vi "Scan.vi"() -> ()   [LabVIEW 2016]
doc: "Ce VI modèle est conçu pour le modèle de conception Gestionnaire de messages dans une file d'attente.\n\nLa boucle de gestion d'événements génère des messages en fonction des actions sur l'interface utilisateur.\n\nLa boucle de gestion de messages traite les messages générés par la boucle de gestion d'événements ou par d'autres messages. Les messages sont des valeurs chaîne ; il est donc facile d'ajouter de nouveaux messages à la structure condition Conditions de messages de la boucle de gestion de messages Chaque cluster Message peut en outre fournir une valeur optionnelle pour Données de message, un variant qui peut être converti aux données requises pour un message spécifique."
uses:
  controls/Enum.ctl
  controls/FPGAVIreferenceTypeDefScanEngine.ctl
  controls/ScanWaveform.ctl
  Course Project/support/Message Queue/Message Cluster.ctl
  <vilib>/Analysis/coordinate.llb/2D Cartesian Coordinate Rotation (Scalar).vi
  <vilib>/rvi/errors/niLvFpgaAdjustHostInterfaceError.vi
  <vilib>/rvi/interface/nirviReadWriteControl/nirviReadWriteControl.xnode
  FPGA Bitfiles/qnmController797_usbRIO_controllerFPGAmu.lvbitx
  <vilib>/regexp/Match Regular Expression.xnode
  Course Project/support/Message Queue/Message Queue.lvlib
  <vilib>/rvi/interface/nirviCloseFPGA/nirviCloseFPGA.xnode
  NiFpgaLv.dll
  <vilib>/Analysis/NI_AALPro.lvlib
  controls/FPGAVIreferenceTypeDef.ctl
  <vilib>/FPGAPlugInAG/USB-7856R OEM/niLvFpga_Close_USB-7856R OEM.vi
panel:
  out "String":string
  in  "Scan Parameters":enum32{"Scan Parameters"}(tab)
  in  "expno":u32
  in  "Exp Folder":string="<date>_exp<expno>"
  in  "Base Folder":path=path "C:/"
  in  "Slow scan axis":bool=TRUE
  out "Speed":dbl format="%#_3pm/s"
  in  "Speed":bool=TRUE
  in  "Lock Scan Lines":bool=TRUE
  in  "Lock Scan Height":bool=TRUE
  in  "Save now":bool
  in  "Auto Save":bool=TRUE
  in  "File name":string="test"
  in  "Scan Parameters":T1={"Width"=1e-09, "Height"=1e-09, "X Offset"=0.0, "Y Offset"=0.0, "Angle"=0.0, "Pixels"=256, "Lines"=256, "Time/Line"=1.0, "Scan Rate"=1.0} {"Scan Rate" format="%#_3pHz"; "Lines" min=2 max=8192 format="%#.0f"; "Pixels" min=2 max=8193 format="%#.0f"; "Height" format="%#.1pm"; "Width" format="%#.1pm"; "Angle" format="%.2f°"; "Y Offset" format="%#_4pm"; "X Offset" format="%#_4pm"; "Time/Line" format="%.2ps"}
  in  "Actions":T2
  # "Scan Parameters"
  # "Frame"
  # "Hz"
  # "s"
  # "Saving"
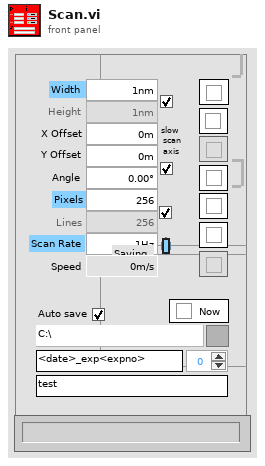
[diagram p1: front panel]
types:
  T1 = cluster{"Width":dbl, "Height":dbl, "X Offset":dbl, "Y Offset":dbl, "Angle":dbl, "Pixels":u16, "Lines":u16, "Time/Line":dbl, "Scan Rate":dbl}
  T2 = cluster{"Frame up":bool, "Frame down":bool, "Flip":bool, "Continuous":bool, "Pause":bool, "Stop":bool, "Move to center":bool}
  T3 = typedef "Message Queue.lvlib/All Message Queues.ctl" = cluster{"IU":refnum<queue>}
  T4 = typedef "Enum.ctl" = enum16{"Init", "Read", "Write"}
  T5 = cluster{"slowMoveWavePts":u16, "slowMoveAccelPts":u16, "moveSpeedSec":dbl}
  T6 = typedef "FPGAVIreferenceTypeDefScanEngine.ctl" = refnum<k20>
  T7 = enum32{"Bad", "Idle", "Run top level", "Running"}
  T8 = typedef "ScanWaveform.ctl" = enum16{"Sine", "Triangle", "Rounded"}
  T9 = cluster{"slowWavePts":u16, "fastWavePts":u16, "slowWaveType":T8, "fastWaveType":T8, "slowRoundPts":u16, "fastRoundPts":u16, "Update Parameters":bool, "Correct Hysteresis":bool, "UpdateFPGA":bool, "Update Graph":bool, "Hysteresis comp?":bool}
  T10 = enum8{"Enabled", "Disabled", "Disabled and Grayed Out"}
  T11 = cluster{"Sensitivity":cluster{"Sens X":dbl, "Sens Y":dbl, "Sens Z":dbl}, "Range":cluster{"Range X":dbl, "Range Y":dbl, "Range Z":dbl}, "HV gain":cluster{"HV gain X":dbl, "HV gain Y":dbl, "HV gain Z":dbl}}
  T12 = typedef "Message Queue.lvlib/Message Cluster.ctl" = cluster{"Message":string, "Données de message":variant}
  T13 = cluster{"slowWavePts":u16, "fastWavePts":u16, "slowWaveType":T8, "fastWaveType":T8, "slowRoundPts":u16, "fastRoundPts":u16, "singleDirectionScan":bool}
  T14 = cluster{"write":bool, "index":u16, "data":fxp<+/-,18,5>}
  T15 = cluster{"calibName":string[], "calibParameters":cluster{"Sensitivity":cluster{"Sens X":dbl, "Sens Y":dbl, "Sens Z":dbl}, "Range":cluster{"Range X":dbl, "Range Y":dbl, "Range Z":dbl}, "HV gain":cluster{"HV gain X":dbl, "HV gain Y":dbl, "HV gain Z":dbl}}[], "calibIndex":i32}
  T16 = cluster{"Sensitivity":cluster{"Sens X":dbl, "Sens Y":dbl, "Sens Z":dbl}, "Range":cluster{"Range X":dbl, "Range Y":dbl, "Range Z":dbl}, "HV gain":cluster{"HV gain X":dbl, "HV gain Y":dbl, "HV gain Z":dbl}}[]
  T17 = cluster{"scanEngineHz":u32, "feedbackHz":u32, "sicmHz":u32, "rampHz":u32}
  T18 = typedef "ScanParametersAllTypeDef.ctl" = cluster{"fastRoundPts":u16, "slowRoundPts":u16, "fastWaveType":T8, "slowWaveType":T8, "fastWavePts":u16, "slowWavePts":u16, "outputRateHz":u32, "yOffset":dbl, "xOffset":dbl, "scanSizeSlow":dbl, "scanSizeFast":dbl, "rotation":dbl, "timePerLine":dbl, "numLines":u16, "pointsPerLine":u32, "scanEnable":bool, "slowMoveWavePts":u16, "slowMoveAccelPts":u16, "moveSpeedSec":dbl, "singleDirectionScan":bool}
  T19 = cluster{"Width":dbl, "Height":dbl, "X Offset":dbl, "Y Offset":dbl, "Angle":dbl, "Pixels/Line":u16, "Lines":u16, "Time/Line":dbl, "Scan Rate":dbl}
  T20 = typedef "FPGAVIreferenceTypeDef.ctl" = refnum<k20>
  T21 = cluster{"fastScanSize":fxp<+,17,1>, "slowScanSize":fxp<+,17,1>, "invertSlowAxis":bool}
  T22 = cluster{"se.p.enable":bool, "se.p.singleDirection":bool, "se.p.haltScan":bool, "se.mot.p.start":bool}
  T23 = cluster{"startFwd":u16, "endFwd":u16, "startBwd":u16, "endBwd":u16, "disableBlanking":bool, "useFineCounter":bool}
  T24 = cluster{"Waveform Shape Fast In":dbl[], "Waveform Shape Slow In":dbl[]}
  T25 = cluster{"outputRate":u16, "fastDecFactor":u16, "outWaveSizeFast":u16, "pplUpsampling":u16, "numLines":u16, "se.p.fastInvDec":fxp<+,22,0>, "se.p.slowUpStep":fxp<+,28,0>, "se.p.outWaveSizeSlow":u16, "blankingMax":u32, "se.p.fastBlanking":cluster{"startFwd":u32, "endFwd":u32, "startBwd":u32, "endBwd":u32, "disableBlanking":bool, "useCoarseCounter":bool}}
  T26 = typedef "ScanWaveform.ctl" = enum16{"Sine Wave", "Triangle Wave", "Rounded Wave"}
  T27 = cluster{"slowWavePts":u16, "fastWavePts":u16, "slowWaveType":T26, "fastWaveType":T26, "slowRoundPts":u16, "fastRoundPts":u16, "Update Parameters":bool, "Correct Hysteresis":bool, "UpdateFPGA":bool, "Update Graph":bool, "Hysteresis comp?":bool}
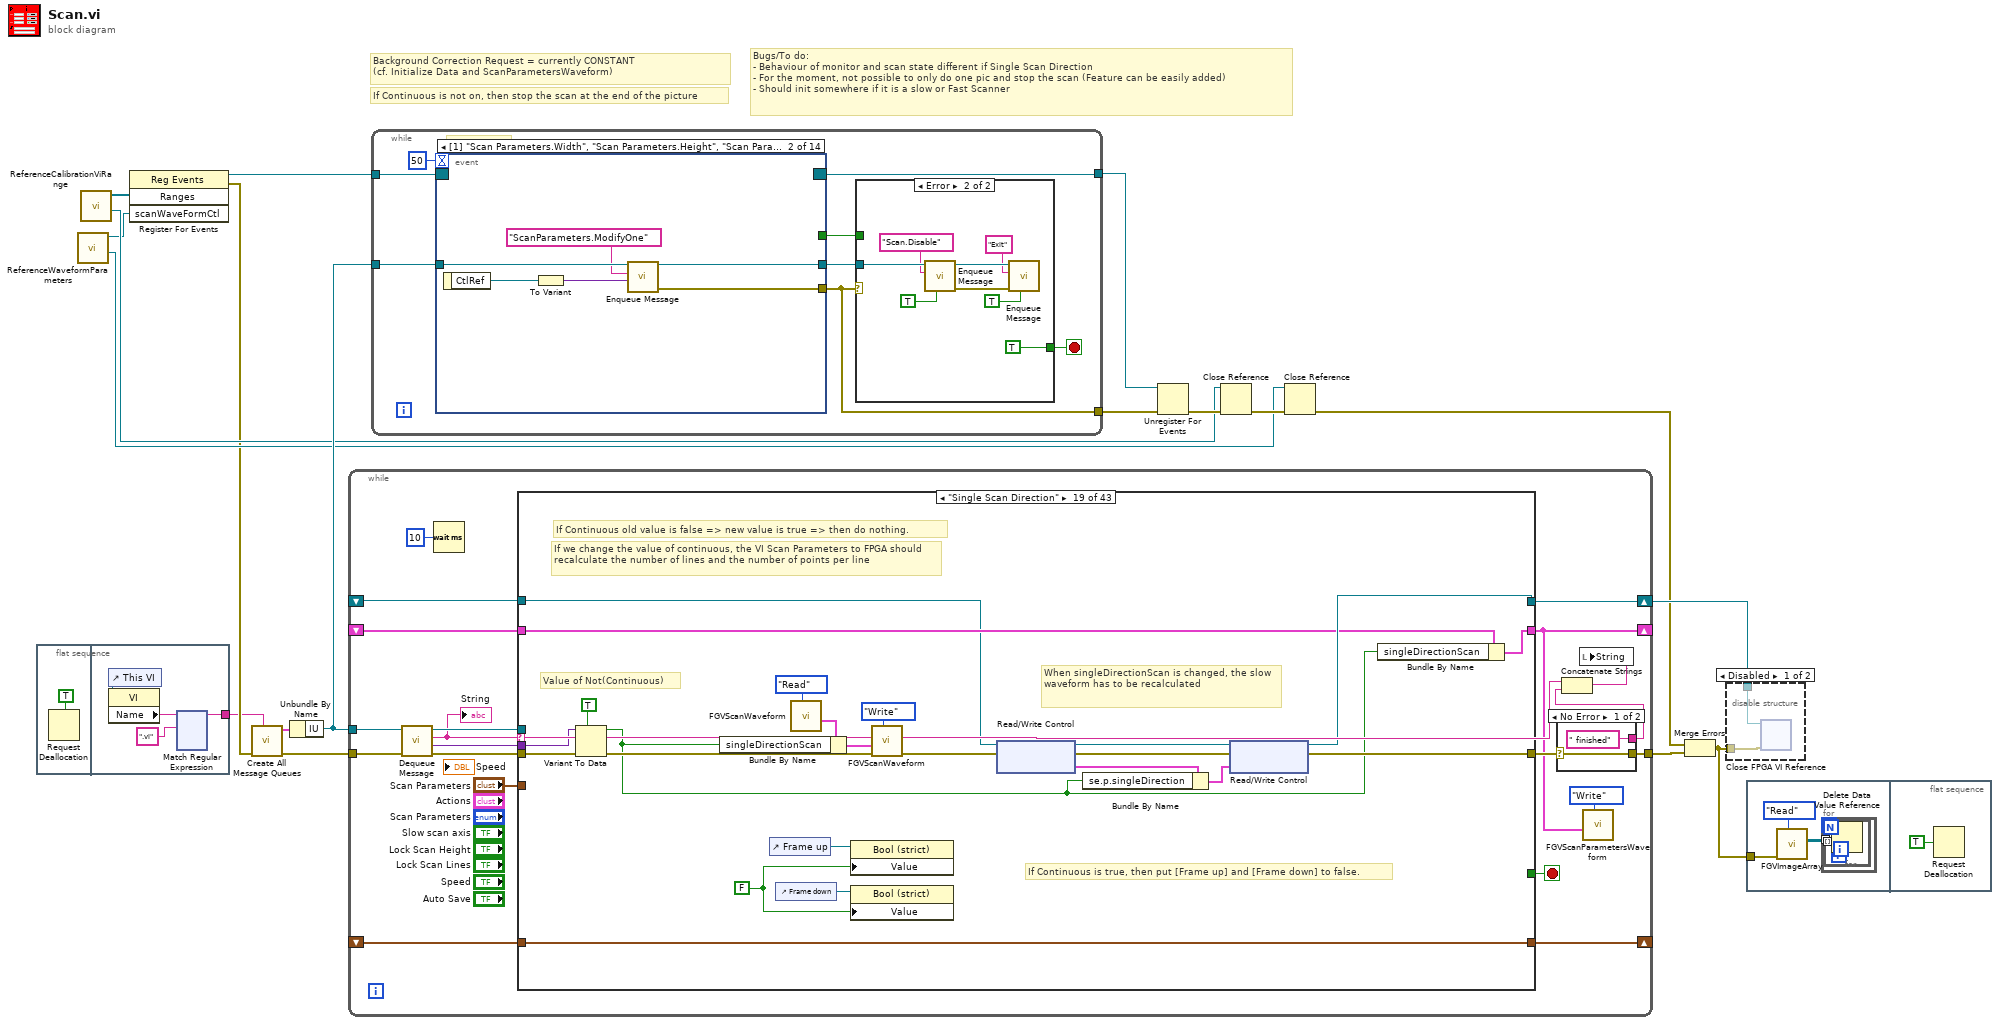
[diagram p0: block diagram]
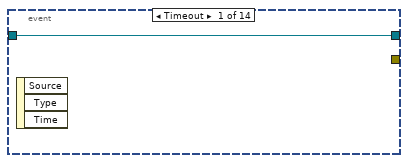
[diagram p4: hidden frame]
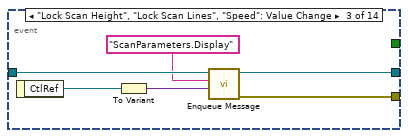
[diagram p5: hidden frame]
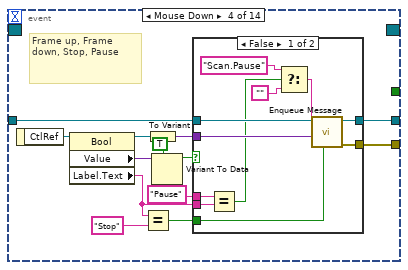
[diagram p6: hidden frame]
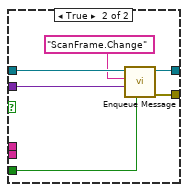
[diagram p7: hidden frame]
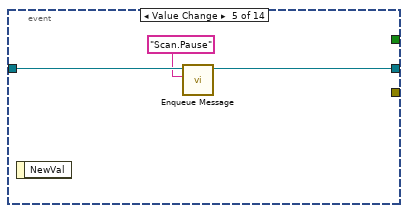
[diagram p8: hidden frame]
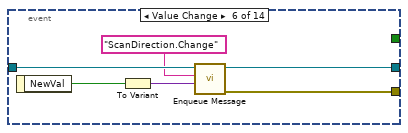
[diagram p9: hidden frame]
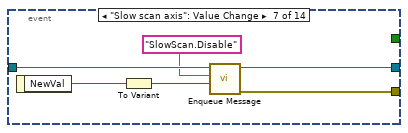
[diagram p10: hidden frame]
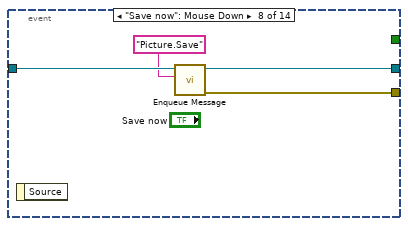
[diagram p11: hidden frame]
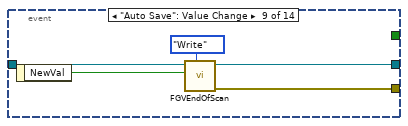
[diagram p12: hidden frame]
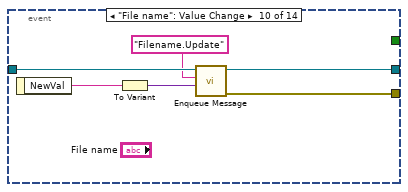
[diagram p13: hidden frame]
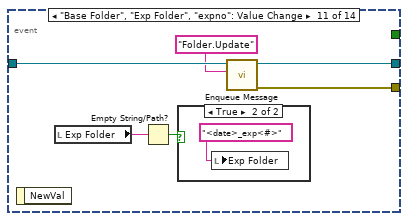
[diagram p14: hidden frame]
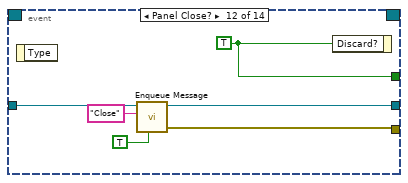
[diagram p16: hidden frame]
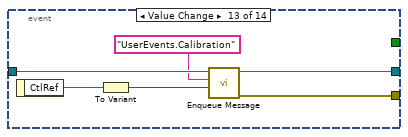
[diagram p17: hidden frame]
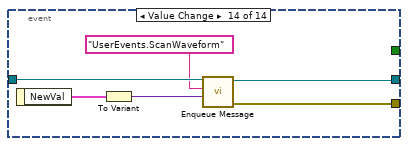
[diagram p18: hidden frame]
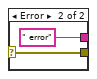
[diagram p19: hidden frame]
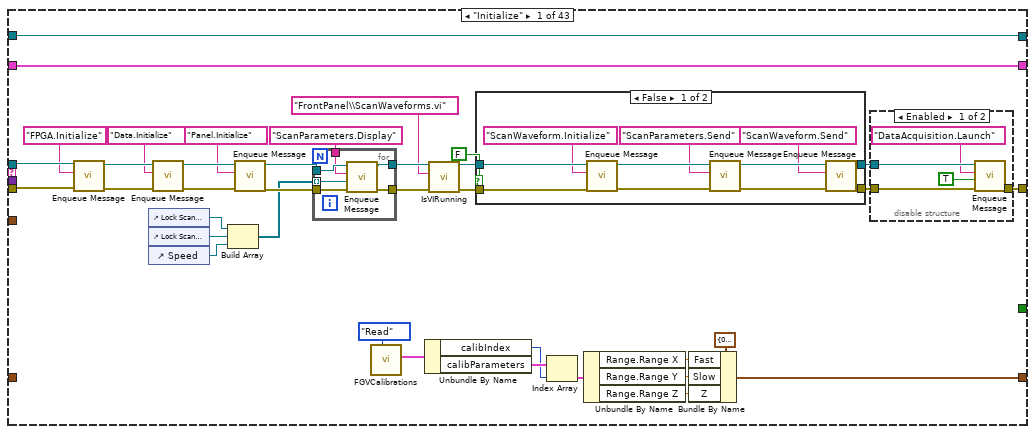
[diagram p20: hidden frame]
diagram:
  # "Bugs/To do:\n- Behaviour of monitor and scan state different if Single Scan Direction\n- For the moment, not possible to only do one pic and stop the scan (Feature can be easily added) \n- Should init somewhere if it is a slow or Fast Scanner"
  # "If Continuous is not on, then stop the scan at the end of the picture"
  # "Background Correction Request = currently CONSTANT\n(cf. Initialize Data and ScanParametersWaveform)"
  n1 = flat-sequence {
    tunnel: [w20] -> w2
    frame #0 {
      n2 = Request Deallocation(TRUE ("flag")) -> ()
    }
    frame #1 {
      n3 = control-ref of="This VI"() -> (w23:refnum<vi>)
      n4 = property class="VI"(reference=w23) -> ("Name"=w22:string)  [unwired: 1 in, 2 out]
      n5 = xnode "Match Regular Expression"("input string"=w22, "regular expression"=".vi") -> ("before match"=w20:string)  [unwired: 4 in, 4 out]
    }
  }
  n6 = call "ReferenceWaveformParameters.vi"() -> ("vi reference"=w5:refnum<vi>, "scanWaveFormCtl"=w7:refnum<vi>)  [unwired: 9 in, 1 out]
  n7 = call "ReferenceCalibrationViRange.vi"() -> ("vi reference"=w8:refnum<vi>, "Ranges"=w12:refnum<vi>[])  [unwired: 8 in, 2 out]
  n8 = register-events(w12, w7) -> (reference out=w11:refnum<event-registration>, error out=w3:errorcluster)  [unwired: 2 in]
  n9 = call "Create All Message Queues.vi"("QueueName"=w2, "ErrorIn"=w3) -> ("ErrorOut"=w18:errorcluster, "MessageQueueOut"=w17:T3)  [unwired: 8 in]
  n10 = Unbundle By Name(w17) -> ("IU"=w15:refnum<queue>)
  n11 = while {
    tunnel: w15 -> [w152]
    shift-right: [w142] -> _
    shift-left: _ -> [w138]
    shift-right: [w144] -> w13
    shift-left: _ -> [w151]
    tunnel: w18 -> [w156]
    tunnel: [w146] -> w16
    shift-right: [w140] -> _
    shift-left: _ -> [w139]
    stop <- w157 stop-if-true
    n12 = call "Dequeue Message.vi"("entrée d'erreur (pas d'erreur)"=w156, "File d'attente de messages"=w152) -> ("sortie d'erreur"=w155:errorcluster, "Données de message"=w154:variant, "Message"=w148:string, "File d'attente de message dup."=w153:refnum<queue>)  [unwired: 6 in]
    "String" <- w148
    n13 = Wait (ms)(milliseconds to wait=u32 10) -> ()  [unwired: 1 out]
    n14 = case "Conditions des messages" shown="\"Single Scan Direction\"" w148 {
      selector: w148 -> [_ _ _ _ _ _ _ _ _ _ _ _ _ _ _ _ _ _ _ _ _ _ _ _ _ _ _ _ _ _ _ _ _ _ _ _ _ _ _ _ _ _ w1429]
      tunnel: w153 -> [w193 _ _ _ _ w411 w430 w463 _ _ _ _ _ _ _ _ w598 w624 _ w739 _ _ w775 _ w880 _ w1114 _ _ _ _ _ _ _ w1312 _ w1342 _ _ _ _ _ _]
      tunnel: w155 -> [w185 w228 w265 w320 w338 w399 w429 w462 w490 w498 w511 w525 w536 w540 w555 w570 w585 w622 w719 w731 w748 w761 w774 w843 w878 w1078 w1108 w1148 w1157 w1162 w1192 w1238 w1272 w1292 w1323 w1330 w1338 w1360 w1373 w1393 w1397 w1405 _]
      tunnel: [w182 w237 w246 w302 w332 w400 w428 w453 w489 w495 w512 w525 w538 w554 w564 w570 w594 w619 w711 w729 w744 w761 w764 w856 w869 w1068 w1099 w1139 w1149 w1162 w1184 w1221 w1271 w1296 w1309 w1330 w1341 w1346 w1369 w1387 w1397 w1402 w1427] -> w147
      tunnel: [_ w239 _ _ _ _ TRUE _ _ _ _ _ _ _ _ _ _ _ _ _ _ _ _ _ _ _ _ _ _ _ _ _ _ _ _ _ _ _ _ _ _ _ _] -> w157
      tunnel: w154 -> [_ _ _ _ w335 _ _ w461 w488 _ _ _ w535 _ _ _ w582 w623 w721 w727 w747 _ w773 _ w879 w1077 w1110 _ _ _ _ _ _ _ _ _ w1336 _ _ _ _ w1404 _]
      tunnel: w138 -> [w190 w242 _ w321 w336 w397 w431 w456 w485 w497 w509 w523 w532 w551 w565 w568 w581 w613 w715 w725 w742 w759 w765 w852 w873 w1086 w1111 w1147 w1156 w1161 w1163 w1241 w1267 w1289 _ w1328 w1339 w1362 w1368 w1392 w1396 w1408 w1424]
      tunnel: [w190 w242 w253 w321 w336 w397 w431 w456 w474 w497 w509 w523 w532 w551 w565 w568 w581 w612 w710 w725 w742 w759 w763 w846 w866 w1070 w1111 w1147 w1156 w1161 w1163 w1241 w1267 w1289 w1313 w1328 w1339 w1343 w1368 w1380 w1396 w1408 w1424] -> w142
      tunnel: [w184 w225 w261 w322 w337 w403 w432 w457 w486 w496 w510 w524 w539 w552 w566 w569 w572 w615 w718 w726 w745 w760 w766 w850 w864 w1082 w1098 w1146 w1155 w1160 w1191 w1239 w1268 w1295 w1326 w1327 w1340 w1347 w1374 w1383 w1395 w1407 w1425] -> w144
      tunnel: w151 -> [w184 _ w261 w322 w337 w403 w432 w457 w486 w496 w510 w524 w539 w552 w566 w569 w573 w616 w705 w726 w746 w760 w766 w851 w865 w1087 w1098 w1146 w1155 w1160 w1170 w1240 w1269 w1294 w1326 w1327 w1340 w1361 w1375 w1388 w1395 w1407 w1425]
      tunnel: "Scan Parameters" -> [_ _ _ _ _ _ _ _ _ _ _ _ _ _ _ _ _ _ _ _ _ _ _ w848 _ w1080 _ _ _ _ _ _ _ _ _ _ _ _ _ _ _ _ _]
      tunnel: [w166 w241 w259 w324 w334 w396 w427 w439 w477 w491 w508 w522 w531 w550 w559 w567 w574 w626 w702 w723 w743 w758 w762 w844 w863 w1073 w1106 w1145 w1154 w1159 w1172 w1237 w1265 w1287 w1325 w1329 w1331 w1358 w1370 w1386 w1394 w1406 w1421] -> w140
      tunnel: w139 -> [_ w241 w259 w324 w334 w396 w427 _ w477 w491 w508 w522 w531 w550 w559 w567 w574 w626 w702 w723 w743 w758 w762 w844 w863 w1073 w1106 w1145 w1154 w1159 w1172 w1237 w1265 w1287 w1325 w1329 w1331 w1358 w1370 w1386 w1394 w1406 w1421]
      frame "Initialize" {
        n15 = call "Enqueue Message.vi"("error in"=w185, "Message"="FPGA.Initialize", "Queue"=w193) -> ("error out"=w189:errorcluster, "Queue dup."=w188:refnum<queue>)  [unwired: 7 in]
        n16 = control-ref of="Lock Scan Height"() -> (w179:refnum<vi>)
        n17 = control-ref of="Lock Scan Lines"() -> (w180:refnum<vi>)
        n18 = control-ref of="Speed"() -> (w181:refnum<vi>)
        n19 = call "Enqueue Message.vi"("error in"=w189, "Message"="Data.Initialize", "Queue"=w188) -> ("error out"=w186:errorcluster, "Queue dup."=w194:refnum<queue>)  [unwired: 7 in]
        n20 = Build Array(w179, w180, w181) -> (w178:refnum<vi>[])
        n21 = call "Enqueue Message.vi"("error in"=w186, "Message"="Panel.Initialize", "Queue"=w194) -> ("error out"=w197:errorcluster, "Queue dup."=w177:refnum<queue>)  [unwired: 7 in]
        n22 = for {
          tunnel: w177 -> [w222]
          tunnel: w178 -> [w221] mode=indexing
          tunnel: [w220] -> w164
          tunnel: w197 -> [w219]
          tunnel: [w218] -> w196
          tunnel: "ScanParameters.Display" ("Message") -> [w217]
          n23 = call "Enqueue Message.vi"("error in"=w219, "Data"=w221, "Message"=w217, "Queue"=w222) -> ("error out"=w220:errorcluster, "Queue dup."=w218:refnum<queue>)  [unwired: 6 in]
        }
        n24 = call "FGVCalibrations.vi"("Enum"=Enum."Read") -> ("calibOut"=w174:T15)  [unwired: 9 in, 1 out]
        n25 = Unbundle By Name(w174) -> ("calibIndex"=w169:i32, "calibParameters"=w173:T16)
        n26 = call "IsVIRunning.vi"("error in (no error)"=w164, "name or relative path"="FrontPanel\\ScanWaveforms.vi") -> ("error out"=w163:errorcluster)  [unwired: 8 in, 1 out]
        n27 = case shown="False" FALSE {
          tunnel: w196 -> [w208 w210]
          tunnel: [w207 w210] -> w195
          tunnel: [w199 w209] -> w183
          tunnel: w163 -> [w198 w209]
          frame False {
            n28 = call "Enqueue Message.vi"("error in"=w198, "Message"="ScanWaveform.Initialize", "Queue"=w208) -> ("error out"=w203:errorcluster, "Queue dup."=w204:refnum<queue>)  [unwired: 7 in]
            n29 = call "Enqueue Message.vi"("error in"=w203, "Message"="ScanParameters.Send", "Queue"=w204) -> ("error out"=w200:errorcluster, "Queue dup."=w206:refnum<queue>)  [unwired: 7 in]
            n30 = call "Enqueue Message.vi"("error in"=w200, "Message"="ScanWaveform.Send", "Queue"=w206) -> ("error out"=w199:errorcluster, "Queue dup."=w207:refnum<queue>)  [unwired: 7 in]
          }
          frame True {
          }
        }
        n31 = Index Array(array=w173, index=w169) -> (element=w170:T11)
        n32 = Unbundle By Name(w170) -> ("Range.Range X"=w172:dbl, "Range.Range Y"=w171:dbl, "Range.Range Z"=w168:dbl)
        n33 = Bundle By Name(cluster=cluster{"Slow":dbl, "Fast":dbl, "Z":dbl} {"Slow"=0.00015, "Fast"=0.00015, "Z"=0.00015} ("Calibration"), "Fast"=w172, "Slow"=w171, "Z"=w168) -> (w166:cluster{"Slow":dbl, "Fast":dbl, "Z":dbl})
        n34 = disable-structure shown="Enabled" {
          disable-tunnel: w195 -> [w215 _]
          disable-tunnel: w183 -> [w213 w216]
          disable-tunnel: [w212 w216] -> w182
          frame Enabled {
            n35 = call "Enqueue Message.vi"("error in"=w213, "Data"=TRUE, "Message"="DataAcquisition.Launch", "Queue"=w215) -> ("error out"=w212:errorcluster)  [unwired: 6 in, 1 out]
          }
          frame Disabled {
          }
        }
      }
      frame "FPGA.Initialize" {
        w224 = cluster{"outputRateHz":u32} {"outputRateHz"=800000}  # ioParams
        (unwired) T5 {"slowMoveWavePts"=1024, "slowMoveAccelPts"=128, "moveSpeedSec"=0.05}  # slowMoveParamsFast
        # "Scan engine output is clocked on base clock"
        # "1 : Scanner J slow\n0,2 : Scanner Fast"
        # "Initialize the Slow mouvment"
        # "ioParameters not Initialized"
        n36 = call "FGVfpgaAdressScanEngine.vi"("Enum"=Enum."Read", "error in"=w228) -> ("error out"=w236:errorcluster, "ioFreqHzOut"=w227:u32, "FPGA.SEout"=w226:T6)  [unwired: 5 in, 2 out]
        n37 = Equal?(x=w226, y=T6 refnum ("FPGAInterfaceOut")) -> (x = y?=w240:bool)
        n38 = Or(x=w236, y=w240) -> (x .or. y?=w239:bool)
        n39 = in-place {
          in-place-border: [w243] -> w230
          in-place-border: w227 -> [w245]
          n40 = in-place-cluster #1(w224) -> ("outputRateHz"=w244:u32)
          n41 = call "corerceFPGAClock.vi"("baseClock"=w245, "requestedFrequency"=w244) -> ("realFrequency"=w243:dbl)  [unwired: 7 in, 2 out]
          n42 = in-place-cluster #1("outputRateHz"=w243) -> (w223:cluster{"outputRateHz":u32})
        }
        n43 = call "FGVSamplingRates.vi"("Enum"=Enum."Read") -> ("samplingRatesOut"=w232:T17)  [unwired: 9 in, 1 out]
        n44 = Bundle By Name(cluster=w232, "scanEngineHz"=w230) -> (w231:T17)
        n45 = call "InitializeSmovement.vi"("error in"=w236, "slowMoveParams"=T5 {"slowMoveWavePts"=131, "slowMoveAccelPts"=30, "moveSpeedSec"=0.05}, "ioParams"=w223, "FPGAInterfaceIn"=w226) -> ("error out"=w237:errorcluster, "FPGAInterfaceOut"=w225:T6)  [unwired: 6 in]
        n46 = call "FGVSamplingRates.vi"("Enum"=Enum."Write", "samplingRatesIn"=w231) -> ()  [unwired: 8 in, 2 out]
      }
      frame "Data.Initialize" {
        # "Replace by Read when the fgv will read a config file"
        # "FGV \nall parameters"
        # "Init Waveform"
        # "Init Scan"
        n47 = local read "Scan Parameters"() -> (w247:T1)
        n48 = call "FGVScanParameters.vi"("Enum"=Enum."Init", "error in"=w265) -> ("error out"=w289:errorcluster)  [unwired: 8 in, 1 out]
        n49 = in-place {
          n50 = in-place-cluster #2(w247) -> ("Width"=w296:dbl, "Height"=w295:dbl, "X Offset"=w294:dbl, "Y Offset"=w293:dbl, "Angle"=w292:dbl, "Pixels"=w291:u16, "Lines"=w290:u16)
          n51 = in-place-cluster #2("Width"=w296, "Height"=w295, "X Offset"=w294, "Y Offset"=w293, "Angle"=w292, "Pixels"=w291, "Lines"=w290) -> (w248:T1)
        }
        n52 = call "FGVScanParametersWaveform.vi"("Enum"=Enum."Init", "error in"=w289) -> ("error out"=w273:errorcluster, "Parameters Out"=w266:T18)  [unwired: 8 in]
        n53 = Unbundle By Name(w266) -> ("outputRateHz"=w267:u32)
        n54 = call "FGVfpgaAdress.vi"("Enum"=Enum."Read") -> ("baseClockOut"=w252:u32)  [unwired: 5 in, 5 out]
        n55 = call "FGVScanWaveform.vi"("Enum"=Enum."Init", "error in"=w273) -> ("error out"=w246:errorcluster, "scanWaveFormCtl Out"=w280:T13)  [unwired: 8 in]
        n56 = call "FGVScanParameters.vi"("Enum"=Enum."Write", "Scan Parameters In"=w248) -> ("Scan Parameters Out"=w249:T19)  [unwired: 8 in, 1 out]
        n57 = Divide(x=w252, y=w267) -> (x/y=w271:dbl)
        n58 = Round Toward -Infinity(1:w271) -> (0:w272:dbl)
        n59 = property on="Continuous" class="Bool (strict)"() -> ("Value"=w251:bool)  [unwired: 2 in, 2 out]
        n60 = Unbundle By Name(w280) -> ("slowWavePts"=w279:u16, "fastWavePts"=w278:u16, "slowWaveType"=w277:T8, "fastWaveType"=w276:T8, "slowRoundPts"=w275:u16, "fastRoundPts"=w274:u16)
        n61 = Unbundle By Name(w249) -> ("Width"=w257:dbl, "Height"=w256:dbl, "X Offset"=w285:dbl, "Y Offset"=w284:dbl, "Angle"=w283:dbl, "Pixels/Line"=w264:u16, "Lines"=w263:u16, "Time/Line"=w282:dbl)
        n62 = In Range and Coerce(upper limit=w272, x=w272, lower limit=43.0) -> (coerced(x)=w269:dbl)  [unwired: 1 out]
        n63 = Divide(x=w252, y=w269) -> (x/y=w268:dbl)
        n64 = Not(x=w251) -> (.not. x?=w262:bool)
        n65 = Divide(x=w257, y=w256) -> (x/y=w258:dbl)
        n66 = property on="Speed" class="DigNum (strict)"("Value"=w258) -> ()  [unwired: 2 in, 2 out]
        n67 = Bundle By Name(cluster=w266, "outputRateHz"=w268, "slowWavePts"=w279, "fastWavePts"=w278, "slowWaveType"=w277, "fastWaveType"=w276, "slowRoundPts"=w275, "fastRoundPts"=w274, "scanSizeFast"=w257, "scanSizeSlow"=w256, "xOffset"=w285, "yOffset"=w284, "rotation"=w283, "pointsPerLine"=w264, "numLines"=w263, "timePerLine"=w282, "scanEnable"=FALSE, "singleDirectionScan"=w262) -> (w254:T18)
        n68 = call "FGVScanParametersWaveform.vi"("Enum"=Enum."Write", "Parameters In"=w254) -> ("Parameters Out"=w253:T18)  [unwired: 8 in, 1 out]
      }
      frame "Panel.Initialize" {
        w298 = "<date>_exp<#>" ("Exp Folder")
        # "Controls in the cluster\n\"Frame...\" which should\nopen on false state"
        # "0,1,3,5,6,7"
        n69 = call "FGVSavingParameters.vi"("Enum"=Enum."Init", "error in"=w320) -> ("filenameOut"=w306:string, "#PicturesSavedOut"=w299:u32, "pathOut"=w305:path)  [unwired: 6 in, 1 out]
        n70 = property on="Base Folder" class="Path"("Value"=w305) -> ()  [unwired: 2 in, 2 out]
        n71 = property on="Actions" class="Clust"() -> ("Controls[]"=w297:refnum<vi>[])  [unwired: 2 in, 2 out]
        n72 = property on="expno" class="DigNum (strict)"("Value"=w299) -> ()  [unwired: 2 in, 2 out]
        n73 = Index Array(array=w297, index #1=0, index #2=1, index #3=2, index #4=4, index #5=5) -> (element #1=w316:refnum<vi>, element #2=w315:refnum<vi>, element #3=w314:refnum<vi>, element #4=w313:refnum<vi>, element #5=w312:refnum<vi>)
        n74 = call "SaveCreatePath.vi"("Exp Folder"=w298, "ExperimentNumber"=w299, "BaseFolder"=w305) -> ("appended path"=w304:path)  [unwired: 7 in, 1 out]
        n75 = property on="Exp Folder" class="Str"("Value"=w298) -> ()  [unwired: 2 in, 2 out]
        n76 = property on="File name" class="Str"("Value"=w306) -> ()  [unwired: 2 in, 2 out]
        n77 = Build Array(w316, w315, w314, w313, w312) -> (w308:refnum<vi>[])
        n78 = for {
          tunnel: w308 -> [w325] mode=indexing
          w330 = refnum<vi> refnum  # Boolean
          n79 = To More Specific Class(target class=w330, reference=w325) -> (specific class reference=w329:refnum<vi>, error out=w328:errorcluster)  [unwired: 1 in]
          n80 = To Variant(anything=FALSE) -> (Variant=w327:variant)
          n81 = property class="Bool"(reference=w329, error in=w328, "Value"=w327) -> ()  [unwired: 2 out]
        }
        n82 = call "FGVSavingParameters.vi"("Enum"=Enum."Write", "filenameIn"=w306, "#PicturesSavedIn"=u32 0, "pathIn"=w304) -> ("error out"=w323:errorcluster)  [unwired: 4 in, 3 out]
        n83 = property on="Auto Save" class="Bool (strict)"() -> ("Value"=w300:bool)  [unwired: 2 in, 2 out]
        n84 = call "FGVEndOfScan.vi"("Enum"=Enum."Write", "error in"=w323, "autoSaveIn"=w300) -> ("error out"=w302:errorcluster)  [unwired: 7 in, 1 out]
      }
      frame "DataAcquisition.Launch" {
        n85 = disable-structure shown="Enabled" {
          disable-tunnel: w338 -> [w352 w395]
          disable-tunnel: w335 -> [w351 _]
          disable-tunnel: [w350 w395] -> w333
          frame Disabled {
            w343 = u8 1 items=["Contact Mode", "ORT", "Aux"] ("fb.i.source")
            n86 = Variant To Data(error in=w352, type=TRUE, Variant=w351) -> (data=w353:bool, error out=w349:errorcluster)
            n87 = call "FGVfpgaAdress.vi"("Enum"=Enum."Read", "error in"=w349) -> ("error out"=w346:errorcluster, "FPGA VI Reference Out"=w347:T20)  [unwired: 4 in, 4 out]
            n88 = xnode "Read/Write Control"("FPGA VI Reference In"=w347, "error in"=w346) -> ("error out"=w345:errorcluster, "fb.i.source"=w344:u8)  [unwired: 1 out]
            n89 = Equal?(x=w344, y=w343) -> (x = y?=w342:bool)
            n90 = Select(t="FrontPanel\\subVIs\\DataAcquisition.vi", s=w342, f="FrontPanel\\subVIs\\DataAcquisitionAux.vi") -> (s? t:f=w339:string)
            n91 = call <vilib>:"Application Directory.vi"() -> ("Application Directory"=w356:path)
            n92 = Build Path(base path=w356, name or relative path=w339) -> (appended path=w357:path)
            n93 = Open VI Reference(vi path=w357, error in (no error)=w345) -> (vi reference=w354:refnum<vi>, error out=w358:errorcluster)  [unwired: 4 in]
            n94 = case "Check the state of the VI: running or closed" shown="False" w353 {
              tunnel: w358 -> [w369 w378]
              tunnel: w354 -> [w362 w387]
              tunnel: [w359 w386] -> w350
              frame False {
                n95 = property class="VI"(reference=w362) -> (reference out=w370:refnum<vi>, "Exec.State"=w364:T7)  [unwired: 1 in, 1 out]
                n96 = Equal?(x=T7."Bad" ("Execution:State"), y=w364) -> (x = y?=w366:bool)
                n97 = Equal?(x=w364, y=T7."Idle" ("Execution:State")) -> (x = y?=w367:bool)
                n98 = Or(x=w366, y=w367) -> (x .or. y?=w368:bool)
                n99 = case shown="False" w368 {
                  tunnel: [w374 w376] -> w361
                  tunnel: [w373 w375] -> w360
                  tunnel: w369 -> [w372 w375]
                  tunnel: w370 -> [w371 w376]
                  frame False {
                    n100 = invoke class="VI" method="Abort VI"(reference=w371, error in=w372) -> (reference out=w374:refnum<vi>, error out=w373:errorcluster)  [unwired: 1 in, 1 out]
                  }
                  frame True {
                  }
                }
                n101 = Close Reference(reference=w361, error in (no error)=w360) -> (error out=w359:errorcluster)
              }
              frame True {
                n102 = property class="VI"(reference=w387, error in=w378) -> (reference out=w385:refnum<vi>, error out=w377:errorcluster, "Exec.State"=w383:T7)
                n103 = Equal?(x=T7."Run top level" ("Execution:State"), y=w383) -> (x = y?=w381:bool)
                n104 = Equal?(x=w383, y=T7."Running" ("Execution:State")) -> (x = y?=w380:bool)
                n105 = Or(x=w381, y=w380) -> (x .or. y?=w379:bool)
                n106 = case shown="False" w379 {
                  tunnel: [w389 w394] -> _
                  tunnel: [w388 w393] -> w386
                  tunnel: w377 -> [w390 w393]
                  tunnel: w385 -> [w391 w394]
                  frame False {
                    n107 = invoke class="VI" method="Run VI"(reference=w391, error in=w390, "Wait until done"=FALSE ("Wait Until Done")) -> (reference out=w389:refnum<vi>, error out=w388:errorcluster)  [unwired: 2 in, 3 out]
                  }
                  frame True {
                  }
                }
              }
            }
          }
          frame Enabled {
          }
        }
        n108 = call "FGVImageArray.vi"("Enum"=Enum."Init", "error in"=w333) -> ("error out"=w332:errorcluster)  [unwired: 8 in, 1 out]
      }
      frame "Close" {
        n109 = disable-structure shown="Disabled" {
          disable-tunnel: w411 -> [w424 w426]
          disable-tunnel: [w423 w426] -> w410
          disable-tunnel: w399 -> [w420 w425]
          disable-tunnel: [w419 w425] -> w398
          frame Disabled {
            n110 = call "Enqueue Message.vi"("Prioritary message"=TRUE ("Message prioritaire ? (F)"), "error in"=w420, "Message"="Settings.Save", "Queue"=w424) -> ("error out"=w419:errorcluster, "Queue dup."=w423:refnum<queue>)  [unwired: 6 in]
          }
          frame Enabled {
          }
        }
        n111 = call "Enqueue Message.vi"("Prioritary message"=TRUE ("Message prioritaire ? (F)"), "error in"=w398, "Message"="Exit", "Queue"=w410) -> ("error out"=w402:errorcluster, "Queue dup."=w408:refnum<queue>)  [unwired: 6 in]
        n112 = call "Enqueue Message.vi"("Prioritary message"=TRUE ("Message prioritaire ? (F)"), "error in"=w402, "Message"="Scan.Disable", "Queue"=w408) -> ("error out"=w401:errorcluster, "Queue dup."=w409:refnum<queue>)  [unwired: 6 in]
        n113 = disable-structure shown="Disabled" {
          disable-tunnel: w409 -> [w417 _]
          disable-tunnel: w401 -> [w413 w418]
          disable-tunnel: [w412 w418] -> w400
          frame Disabled {
            n114 = call "Enqueue Message.vi"("Prioritary message"=TRUE ("Message prioritaire ? (F)"), "error in"=w413, "Data"=FALSE ("Message prioritaire ? (F)"), "Message"="DataAcquisition.Launch", "Queue"=w417) -> ("error out"=w412:errorcluster)  [unwired: 5 in, 1 out]
          }
          frame Enabled {
          }
        }
      }
      frame "Exit" {
        n115 = disable-structure shown="Disabled" {
          frame Disabled {
            n116 = call <vilib>:"Three Button Dialog.vi"("Right Button Text (\"Cancel\")"="Stop the scan" ("Right Button Text (\"Cancel\")"), "Center Button Text (\"No\")"="Close the window only" ("Center Button Text (\"No\")"), "Left Button Text (\"Yes\")"="Yes to all" ("Left Button Text (\"Yes\")"), "message"="Do you want to close the window and stop the scan?") -> ()  [unwired: 7 in, 1 out]
          }
          frame Enabled {
          }
        }
        n117 = Release Queue(queue=w430, error in (no error)=w429) -> (error out=w428:errorcluster)  [unwired: 1 in, 2 out]
      }
      frame "UserEvents.Calibration" {
        n118 = Variant To Data(error in=w462, type=refnum<vi> refnum ("CtlRef"), Variant=w461) -> (data=w459:refnum<vi>, error out=w458:errorcluster)
        n119 = property class="Ctl"(reference=w459, error in=w458) -> (error out=w464:errorcluster, "Label.Text"=w455:string, "Value"=w451:variant)  [unwired: 1 out]
        n120 = call "FGVCalibrations.vi"("Enum"=Enum."Read") -> ("calibOut"=w448:T15)  [unwired: 9 in, 1 out]
        n121 = Variant To Data(error in=w464, type=0.0, Variant=w451) -> (data=w449:dbl, error out=w450:errorcluster)
        n122 = Unbundle By Name(w448) -> ("calibIndex"=w446:i32, "calibParameters"=w447:T16)
        n123 = Index Array(array=w447, index=w446) -> (element=w440:T11)
        n124 = case shown="\"Range X\"" w455 {
          tunnel: w450 -> [_ _ _]
          tunnel: w449 -> [w466 w468 w471]
          tunnel: w440 -> [w467 w469 w473]
          tunnel: [w465 w470 w472] -> w438
          frame "Range Y", Default {
            n125 = Bundle By Name(cluster=w467, "Range.Range Y"=w466) -> (w465:T11)
          }
          frame "Range Z" {
            n126 = Bundle By Name(cluster=w469, "Range.Range Z"=w468) -> (w470:T11)
          }
          frame "Range X" {
            n127 = Bundle By Name(cluster=w473, "Range.Range X"=w471) -> (w472:T11)
          }
        }
        n128 = Unbundle By Name(w438) -> ("Range.Range X"=w443:dbl, "Range.Range Y"=w442:dbl, "Range.Range Z"=w441:dbl)
        n129 = call "Enqueue Message.vi"("Data"=w438, "Message"="ScanParameters.WritetoFPGA", "Queue"=w463) -> ("error out"=w453:errorcluster)  [unwired: 7 in, 1 out]
        n130 = Bundle By Name(cluster=cluster{"Slow":dbl, "Fast":dbl, "Z":dbl} {"Slow"=0.00015, "Fast"=0.00015, "Z"=0.00015} ("Calibration"), "Fast"=w443, "Slow"=w442, "Z"=w441) -> (w439:cluster{"Slow":dbl, "Fast":dbl, "Z":dbl})
      }
      frame "UserEvents.ScanWaveform" {
        n131 = Variant To Data(error in=w490, type=T9 {"slowWavePts"=0, "fastWavePts"=0, "slowWaveType"=enum."Sine", "fastWaveType"=enum."Sine", "slowRoundPts"=0, "fastRoundPts"=0, "Update Parameters"=FALSE, "Correct Hysteresis"=FALSE, "UpdateFPGA"=FALSE, "Update Graph"=FALSE, "Hysteresis comp?"=FALSE} ("NewVal"), Variant=w488) -> (data=w484:T9, error out=w489:errorcluster)
        n132 = Unbundle By Name(w484) -> ("fastRoundPts"=w483:u16, "slowRoundPts"=w482:u16, "fastWaveType"=w481:T8, "slowWaveType"=w480:T8, "fastWavePts"=w479:u16, "slowWavePts"=w478:u16)
        n133 = Bundle By Name(cluster=w485, "fastRoundPts"=w483, "slowRoundPts"=w482, "fastWaveType"=w481, "slowWaveType"=w480, "fastWavePts"=w479, "slowWavePts"=w478) -> (w475:T18)
        n134 = call "FGVScanParametersWaveform.vi"("Enum"=Enum."Write", "Parameters In"=w475) -> ("Parameters Out"=w474:T18)  [unwired: 8 in, 1 out]
      }
      frame "Settings.Load" {
        # "2"
        # "1"
        n135 = call <vilib>:"Application Directory.vi"() -> ("Application Directory"=w493:path)
        n136 = Build Path(base path=w493, name or relative path="Settings.ini" ("file (use dialog)")) -> (appended path=w492:path)
        n137 = Read from Text File(file (use dialog)=w492, error in=w498) -> (text=w502:string, error out=w503:errorcluster)  [unwired: 2 in, 2 out]
        n138 = Unflatten From String(type=cluster{string, variant}[] [], binary string=w502, error in (no error)=w503) -> (value=w500:cluster{string, variant}[], error out=w495:errorcluster)  [unwired: 2 in, 1 out]
        n139 = control-ref of="This VI"() -> (w501:refnum<vi>)
        n140 = for {
          tunnel: w501 -> [w507]
          tunnel: w500 -> [w506] mode=indexing
          # "3"
          n141 = Unbundle(w506) -> (w504:string, w505:variant)
          n142 = invoke class="VI" method="Ctrl Val.Set"(reference=w507, "Control Name"=w504, "Value"=w505) -> ()  [unwired: 2 in, 5 out]
        }
      }
      frame "Settings.Save" {
        # "3"
        # "2"
        # "1"
        n143 = control-ref of="This VI"() -> (w521:refnum<vi>)
        n144 = invoke class="VI" method="Ctrl Val.Get All"(reference=w521, error in=w511, "Controls"=TRUE) -> (error out=w517:errorcluster, "Get All Control Values Variant"=w516:cluster{"Name":string, "Variant Data":variant}[])  [unwired: 1 in, 2 out]
        n145 = Flatten To String(anything=w516, error in (no error)=w517) -> (data string=w518:string, error out=w519:errorcluster)  [unwired: 2 in, 1 out]
        n146 = Write to Text File(text=w518, error in=w519) -> (refnum out=w514:refnum<file>, error out=w515:errorcluster)  [unwired: 2 in, 1 out]
        n147 = Close File(refnum=w514, error in=w515) -> (error out=w513:errorcluster)  [unwired: 1 out]
        n148 = call <vilib>:"Simple Error Handler.vi"("error in (no error)"=w513) -> ("error out"=w512:errorcluster)  [unwired: 4 in, 4 out]
      }
      frame " ---------- Saving  ---------- " {
      }
      frame "Filename.Update" {
        n149 = Variant To Data(error in=w536, type="", Variant=w535) -> (data=w533:string, error out=w529:errorcluster)
        n150 = call "FGVSavingParameters.vi"("Enum"=Enum."Read", "error in"=w529) -> ("error out"=w528:errorcluster, "#PicturesSavedOut"=w526:u32, "pathOut"=w527:path)  [unwired: 6 in, 1 out]
        n151 = call "FGVSavingParameters.vi"("Enum"=Enum."Write", "error in"=w528, "filenameIn"=w533, "#PicturesSavedIn"=w526, "pathIn"=w527) -> ("error out"=w538:errorcluster)  [unwired: 3 in, 3 out]
      }
      frame "Folder.Update" {
        # "There is no update of the date from one day to another except if updated folder through this condition"
        # "Creates a new Folder with the current date"
        n152 = call "SaveCreatePath.vi"("error in"=w540, "Exp Folder"="Exp Folder", "ExperimentNumber"="expno", "BaseFolder"="Base Folder") -> ("error out"=w541:errorcluster, "appended path"=w542:path)  [unwired: 6 in]
        n153 = call "FGVSavingParameters.vi"("Enum"=Enum."Read", "error in"=w541) -> ("error out"=w548:errorcluster, "filenameOut"=w546:string, "#PicturesSavedOut"=w547:u32)  [unwired: 6 in, 1 out]
        n154 = call "FGVSavingParameters.vi"("Enum"=Enum."Write", "error in"=w548, "filenameIn"=w546, "#PicturesSavedIn"=w547, "pathIn"=w542) -> ("error out"=w554:errorcluster)  [unwired: 3 in, 3 out]
      }
      frame "Picture.Save" {
        n155 = call "FGVSavingParameters.vi"("Enum"=Enum."Read") -> ("filenameOut"=w557:string, "pathOut"=w556:path)  [unwired: 7 in, 2 out]
        n156 = Get Date/Time In Seconds() -> (seconds since 1Jan1904=w562:timestamp)
        n157 = call "Save.vi"("current time"=w562, "base path"=w556, "error in"=w555, "Filename"=w557) -> ("error out"=w561:errorcluster)  [unwired: 6 in, 1 out]
        n158 = call <vilib>:"Clear Errors.vi"("error in (no error)"=w561) -> ("error out"=w560:errorcluster)  [unwired: 5 in, 1 out]
        n159 = property on="Save now" class="Bool (strict)"(error in=w560, "Value"=FALSE ("Save now")) -> (error out=w564:errorcluster)  [unwired: 1 in, 1 out]
      }
      frame "-------- Scan Direction --------" {
      }
      frame "ScanDirection.Change" {
        # "Change the Scan direction from Single direction to Continuous?"
        # "Stops the Scan"
        n160 = Variant To Data(error in=w585, type=TRUE, Variant=w582) -> (data=w579:bool, error out=w584:errorcluster)
        n161 = xnode "Read/Write Control"("FPGA VI Reference In"=w573, "error in"=w584) -> ("FPGA VI Reference Out"=w572:T6, "error out"=w595:errorcluster, "se.p.modes.se.p.enable"=w586:bool)
        n162 = case shown="True" w586 {
          tunnel: [w601 w604] -> w588
          tunnel: w595 -> [w601 w603]
          tunnel: w598 -> [w600 w606]
          tunnel: [w600 w602] -> w597
          frame False {
          }
          frame True {
            n163 = call "Enqueue Message.vi"("error in"=w603, "Message"="Scan.Disable", "Queue"=w606) -> ("error out"=w604:errorcluster, "Queue dup."=w602:refnum<queue>)  [unwired: 7 in]
          }
        }
        n164 = Not(x=w579) -> (.not. x?=w580:bool)
        n165 = To Variant(anything=w580) -> (Variant=w571:variant)
        n166 = call "Enqueue Message.vi"("error in"=w588, "Data"=w571, "Message"="Single Scan Direction", "Queue"=w597) -> ("error out"=w587:errorcluster, "Queue dup."=w596:refnum<queue>)  [unwired: 6 in]
        n167 = call "Enqueue Message.vi"("error in"=w587, "Message"="ScanWaveform.Initialize", "Queue"=w596) -> ("error out"=w577:errorcluster, "Queue dup."=w578:refnum<queue>)  [unwired: 7 in]
        n168 = call "Enqueue Message.vi"("error in"=w577, "Message"="ScanWaveform.Send", "Queue"=w578) -> ("error out"=w589:errorcluster, "Queue dup."=w599:refnum<queue>)  [unwired: 7 in]
        n169 = call "Enqueue Message.vi"("error in"=w589, "Message"="ScanParameters.Send", "Queue"=w599) -> ("error out"=w591:errorcluster, "Queue dup."=w592:refnum<queue>)  [unwired: 7 in]
        n170 = case shown="True" w586 {
          tunnel: w591 -> [w607 w609]
          tunnel: [w607 w608] -> w594
          tunnel: w592 -> [_ w611]
          frame False {
          }
          frame True {
            n171 = call "Enqueue Message.vi"("error in"=w609, "Message"="Scan.Enable", "Queue"=w611) -> ("error out"=w608:errorcluster)  [unwired: 7 in, 1 out]
          }
        }
      }
      frame "ScanFrame.Change" {
        # "Label of the button clicked"
        # "- If Frame up pressed: disactivate the scan, send an negative height, reenable the scan\n- If Frame down pressed: disactivate the scan, send a positive height, reenable the scan\n- If Flip is pressed: for the moment IT DOESNT WORK because the tip goes to origin when disabled\n- If Continuous is pressed, reverse scan at the end of the scan except if Frame up or Frame down is pressed\n- If Stop is pressed, disable scan"
        n172 = Variant To Data(error in=w622, type=refnum<vi> refnum ("CtlRef"), Variant=w623) -> (data=w621:refnum<vi>, error out=w614:errorcluster)
        n173 = property class="Bool"(reference=w621, error in=w614) -> (error out=w625:errorcluster, "Label.Text"=w618:string)  [unwired: 1 out]
        n174 = case shown="\"Frame down\", \"Frame up\"" w618 {
          selector: w618 -> [_ w675 _ _]
          tunnel: [w631 w671 w687 w696] -> w619
          tunnel: w625 -> [w629 w638 w690 w694]
          tunnel: w624 -> [w632 w679 w692 w698]
          tunnel: "Frame up" -> [_ w673 _ _]
          tunnel: w616 -> [w628 w668 w688 w695]
          tunnel: [w628 w640 w688 w695] -> w615
          tunnel: w613 -> [w627 w642 w683 w693]
          tunnel: [w627 w642 w683 w693] -> w612
          tunnel: w626 -> [_ w643 _ _]
          frame "", Default {
            n175 = call "Enqueue Message.vi"("error in"=w629, "Message"="Default", "Queue"=w632) -> ("error out"=w631:errorcluster)  [unwired: 7 in, 1 out]
          }
          frame "Frame down", "Frame up" {
            w672 = FALSE ("Value")
            n176 = Equal?(x=w675, y=w673) -> (x = y?=w669:bool)
            n177 = call "ConvertScanSizeto01.vi"("error in (no error)"=w638, "Parameters In"=w642, "Calibration"=w643) -> ("error out"=w682:errorcluster, "Parameters Out"=w641:T18)  [unwired: 4 in, 3 out]
            n178 = Unbundle By Name(w641) -> ("xOffset"=w653:dbl, "scanSizeFast"=w656:dbl, "scanSizeSlow"=w654:dbl, "yOffset"=w652:dbl, "rotation"=w648:dbl)
            n179 = Select(t=TRUE, s=w669, f=FALSE) -> (s? t:f=w681:bool)
            n180 = xnode "Read/Write Control"("FPGA VI Reference In"=w668, "error in"=w682) -> ("FPGA VI Reference Out"=w667:T6, "error out"=w666:errorcluster, "se.p.scanSize"=w665:T21)
            n181 = expression code="-(x/180.0)*pi" "degrees to radians"(w648) -> (w636:dbl)
            n182 = Negate(x=w656) -> (-x=w647:dbl)
            n183 = Negate(x=w654) -> (-x=w645:dbl)
            n184 = Bundle By Name(cluster=w665, "invertSlowAxis"=w681) -> (w637:T21)
            n185 = Select(t=w654, s=w681, f=w645) -> (s? t:f=w655:dbl)
            n186 = call-poly <vilib>:"2D Cartesian Coordinate Rotation.vi"("theta"=w636, "y"=w655, "x"=w647) -> ("y out"=w651:dbl, "x out"=w646:dbl)  [unwired: 6 in, 1 out]
            n187 = Add(x=w653, y=w646) -> (x+y=w649:dbl)
            n188 = Add(x=w651, y=w652) -> (x+y=w650:dbl)
            n189 = Bundle By Name(cluster=cluster{"x":fxp<+/-,16,1>, "y":fxp<+/-,16,1>} {"x"=0.0, "y"=0.0} ("moveToPoint"), "x"=w649, "y"=w650) -> (w644:cluster{"x":fxp<+/-,16,1>, "y":fxp<+/-,16,1>})
            n190 = xnode "Read/Write Control"("FPGA VI Reference In"=w667, "error in"=w666, "se.p.scanSize"=w637, "se.mot.p.target"=w644) -> ("FPGA VI Reference Out"=w640:T6, "error out"=w660:errorcluster)
            n191 = call "FGVWaveformShape.vi"("Enum"=Enum."Read", "error in"=w660) -> ("error out"=w661:errorcluster, "Waveform Shape Slow Out"=w658:dbl[], "Waveform Shape Fast Out"=w659:dbl[])  [unwired: 5 in, 2 out]
            n192 = call "FGVWaveformShape.vi"("Framing up? (down: f) In"=w681, "Enum"=Enum."Write", "error in"=w661, "Waveform Shape Slow In"=w658, "Waveform Shape Fast In"=w659) -> ("error out"=w635:errorcluster)  [unwired: 2 in, 4 out]
            n193 = call "FGVLineIndexElementsRemaining.vi"("Enum"=Enum."Init", "error in"=w635) -> ("error out"=w634:errorcluster)  [unwired: 8 in, 1 out]
            n194 = call "Enqueue Message.vi"("error in"=w634, "Message"="Scan.Disable", "Queue"=w679) -> ("error out"=w674:errorcluster, "Queue dup."=w680:refnum<queue>)  [unwired: 7 in]
            n195 = call "Enqueue Message.vi"("error in"=w674, "Message"="Scan.Enable", "Queue"=w680) -> ("error out"=w664:errorcluster)  [unwired: 7 in, 1 out]
            n196 = property on="Frame up" class="Bool (strict)"(error in=w664, "Value"=w672) -> (error out=w670:errorcluster)  [unwired: 1 in, 1 out]
            n197 = property on="Frame down" class="Bool (strict)"(error in=w670, "Value"=w672) -> (error out=w671:errorcluster)  [unwired: 1 in, 1 out]
          }
          frame "Stop" {
            (unwired) "You clicked on Stop. The tip goes to the origin of the scan" ("Message")
            n198 = call "Enqueue Message.vi"("Prioritary message"=TRUE ("Message prioritaire ? (F)"), "error in"=w690, "Message"="Scan.Disable", "Queue"=w692) -> ("error out"=w686:errorcluster)  [unwired: 6 in, 1 out]
            n199 = Unbundle By Name(w686) -> ("status"=w684:bool)
            n200 = property on="Frame up" class="Bool (strict)"(error in=w686, "Value"=w684) -> (error out=w685:errorcluster)  [unwired: 1 in, 1 out]
            n201 = property on="Frame down" class="Bool (strict)"(error in=w685, "Value"=w684) -> (error out=w687:errorcluster)  [unwired: 1 in, 1 out]
          }
          frame "Pause" {
            n202 = call "Enqueue Message.vi"("error in"=w694, "Message"="Scan.Pause", "Queue"=w698) -> ("error out"=w696:errorcluster)  [unwired: 7 in, 1 out]
          }
        }
      }
      frame "Single Scan Direction" {
        w699 = FALSE ("Value")
        # "When singleDirectionScan is changed, the slow waveform has to be recalculated"
        # "If we change the value of continuous, the VI Scan Parameters to FPGA should recalculate the number of lines and the number of points per line"
        # "Value of Not(Continuous)"
        # "If Continuous old value is false => new value is true => then do nothing."
        # "If Continuous is true, then put [Frame up] and [Frame down] to false."
        n203 = Variant To Data(error in=w719, type=TRUE, Variant=w721) -> (data=w703:bool, error out=w717:errorcluster)
        n204 = control-ref of="Frame up"() -> (w701:refnum<vi>)
        n205 = control-ref of="Frame down"() -> (w700:refnum<vi>)
        n206 = call "FGVScanWaveform.vi"("Enum"=Enum."Read") -> ("scanWaveFormCtl Out"=w713:T13)  [unwired: 9 in, 1 out]
        n207 = Bundle By Name(cluster=w713, "singleDirectionScan"=w703) -> (w712:T13)
        n208 = property class="Bool (strict)"(reference=w701, "Value"=w699) -> ()  [unwired: 1 in, 2 out]
        n209 = property class="Bool (strict)"(reference=w700, "Value"=w699) -> ()  [unwired: 1 in, 2 out]
        n210 = call "FGVScanWaveform.vi"("Enum"=Enum."Write", "error in"=w717, "scanWaveFormCtl In"=w712) -> ("error out"=w707:errorcluster)  [unwired: 7 in, 1 out]
        n211 = xnode "Read/Write Control"("FPGA VI Reference In"=w705, "error in"=w707) -> ("FPGA VI Reference Out"=w704:T6, "error out"=w706:errorcluster, "se.p.modes"=w708:T22)
        n212 = Bundle By Name(cluster=w708, "se.p.singleDirection"=w703) -> (w709:T22)
        n213 = xnode "Read/Write Control"("FPGA VI Reference In"=w704, "error in"=w706, "se.p.modes"=w709) -> ("FPGA VI Reference Out"=w718:T6, "error out"=w711:errorcluster)
        n214 = Bundle By Name(cluster=w715, "singleDirectionScan"=w703) -> (w710:T18)
      }
      frame "SlowScan.Disable" {
        n215 = Variant To Data(error in=w731, type=TRUE ("NewVal"), Variant=w727) -> (data=w724:bool, error out=w730:errorcluster)
        n216 = call "Enqueue Message.vi"("error in"=w730, "Message"="Scan.Enable", "Queue"=w739) -> ("error out"=w736:errorcluster, "Queue dup."=w737:refnum<queue>)  [unwired: 7 in]
        n217 = To Variant(anything=w724) -> (Variant=w722:variant)
        n218 = call "Enqueue Message.vi"("error in"=w736, "Data"=w722, "Message"="SlowScanAxis.Disable", "Queue"=w737) -> ("error out"=w734:errorcluster, "Queue dup."=w733:refnum<queue>)  [unwired: 6 in]
        n219 = call "Enqueue Message.vi"("error in"=w734, "Message"="Scan.Disable", "Queue"=w733) -> ("error out"=w729:errorcluster)  [unwired: 7 in, 1 out]
      }
      frame "SlowScanAxis.Disable" {
        # "OR we nullify the waveform, or we define the number of lines to 1 or we define the Y size to the size of a line"
        n220 = Variant To Data(error in=w748, type=TRUE, Variant=w747) -> (data=w741:bool, error out=w752:errorcluster)
        n221 = in-place {
          in-place-border: w741 -> [w754]
          n222 = in-place-cluster #3(w742) -> ("scanSizeSlow"=w756:dbl, "numLines"=w753:u16)
          n223 = Divide(x=w756, y=w753) -> (x/y=w757:dbl)
          n224 = Select(t=w756, s=w754, f=w757) -> (s? t:f=w755:dbl)
          n225 = in-place-cluster #3("scanSizeSlow"=w755, "numLines"=w753) -> (w740:T18)
        }
        n226 = call "ConvertScanSizeto01.vi"("error in (no error)"=w752, "Parameters In"=w740, "Calibration"=w743) -> ("error out"=w751:errorcluster, "Parameters Out"=w750:T18)  [unwired: 4 in, 3 out]
        n227 = call "ScanparametersToFPGA.vi"("error in"=w751, "Parameters In"=w750, "FPGAIn"=w746) -> ("error out"=w744:errorcluster, "FPGAOut"=w745:T6)  [unwired: 4 in, 3 out]
      }
      frame "------- Scan Parameters --------" {
      }
      frame "ScanParameters.Display" {
        # "and with the display or either Scan Rate or Time/Lines"
        # "Plays with the lockers of Scan Size and Scan Points"
        n228 = Variant To Data(error in=w774, type=refnum<vi> refnum ("CtlRef"), Variant=w773) -> (data=w768:refnum<vi>, error out=w772:errorcluster)
        n229 = property class="Bool (strict)"(reference=w768, error in=w772) -> (error out=w770:errorcluster, "Label.Text"=w771:string, "Value"=w767:bool)  [unwired: 1 out]
        n230 = case shown="\"Speed\"" w771 {
          tunnel: w767 -> [w790 w805 w823 _]
          tunnel: w770 -> [w786 w803 w830 w842]
          tunnel: [w777 w795 w829 w842] -> w764
          tunnel: w775 -> [_ _ _ _]
          tunnel: w765 -> [w784 w800 w820 w841]
          tunnel: [w783 w801 w820 w841] -> w763
          frame "Lock Scan Height" {
            n231 = control-ref of="Height"() -> (w788:refnum<vi>)
            n232 = control-ref of="Width"() -> (w787:refnum<vi>)
            n233 = property class="DigNum (strict)"(reference=w787, error in=w786) -> (error out=w785:errorcluster, "Value"=w776:dbl)  [unwired: 1 out]
            n234 = Select(t=T10."Disabled and Grayed Out" ("Disabled"), s=w790, f=T10."Enabled" ("Disabled")) -> (s? t:f=w789:T10)
            n235 = property class="DigNum (strict)"(reference=w788, error in=w785, "Value"=w776, "DisabledEnum"=w789) -> (error out=w779:errorcluster)  [unwired: 1 out]
            n236 = Bundle By Name(cluster=w784, "scanSizeSlow"=w776) -> (w783:T18)
            n237 = call "FGVScanParameters.vi"("Enum"=Enum."Read", "error in"=w779) -> ("error out"=w793:errorcluster, "Scan Parameters Out"=w781:T19)  [unwired: 8 in]
            n238 = Bundle By Name(cluster=w781, "Height"=w776) -> (w782:T19)
            n239 = call "FGVScanParameters.vi"("Enum"=Enum."Write", "error in"=w793, "Scan Parameters In"=w782) -> ("error out"=w777:errorcluster)  [unwired: 7 in, 1 out]
          }
          frame "Lock Scan Lines" {
            n240 = control-ref of="Lines"() -> (w806:refnum<vi>)
            n241 = control-ref of="Pixels"() -> (w802:refnum<vi>)
            n242 = property class="DigNum (strict)"(reference=w802, error in=w803) -> (error out=w804:errorcluster, "Value"=w794:u16)  [unwired: 1 out]
            n243 = Select(t=T10."Disabled and Grayed Out" ("Disabled"), s=w805, f=T10."Enabled" ("Disabled")) -> (s? t:f=w808:T10)
            n244 = property class="DigNum (strict)"(reference=w806, error in=w804, "Value"=w794, "DisabledEnum"=w808) -> (error out=w810:errorcluster)  [unwired: 1 out]
            n245 = Bundle By Name(cluster=w800, "numLines"=w794) -> (w801:T18)
            n246 = property on="Pixels" class="DigNum (strict)"("Val(Sgnl)"=w794) -> ()  [unwired: 2 in, 2 out]
            n247 = call "FGVScanParameters.vi"("Enum"=Enum."Read") -> ("Scan Parameters Out"=w797:T19)  [unwired: 9 in, 1 out]
            n248 = property on="Lines" class="DigNum (strict)"("Val(Sgnl)"=w794) -> ()  [unwired: 2 in, 2 out]
            n249 = Bundle By Name(cluster=w797, "Lines"=w794) -> (w799:T19)
            n250 = call "FGVScanParameters.vi"("Enum"=Enum."Write", "error in"=w810, "Scan Parameters In"=w799) -> ("error out"=w795:errorcluster)  [unwired: 7 in, 1 out]
          }
          frame "Speed" {
            # "Scan Rate"
            # "Time/Line"
            # "Boolean text"
            n251 = control-ref of="Time/Line"() -> (w826:refnum<vi>)
            n252 = control-ref of="Scan Rate"() -> (w824:refnum<vi>)
            n253 = case shown="True" w823 {
              tunnel: w830 -> [w831 w836]
              tunnel: [w831 w836] -> w829
              tunnel: [w833 w840] -> w828
              tunnel: w824 -> [w833 w840]
              tunnel: [w832 w839] -> w827
              tunnel: w826 -> [w832 w839]
              tunnel: [FALSE TRUE] -> w821
              tunnel: [TRUE FALSE] -> w825
              frame False {
                # "Scan Rate \nFalse"
              }
              frame True {
                # "Time/Line\nTrue"
              }
            }
            n254 = property class="DigNum (strict)"(reference=w828, "Visible"=w821) -> ("Value"=w816:dbl)  [unwired: 1 in, 2 out]
            n255 = property class="DigNum (strict)"(reference=w827, "Visible"=w825) -> ("Value"=w818:dbl)  [unwired: 1 in, 2 out]
            n256 = Unbundle By Name(w820) -> ("scanSizeFast"=w817:dbl)
            n257 = Divide(x=w817, y=w818) -> (x/y=w815:dbl)
            n258 = Compound Arithmetic op=MULTIPLY(2.0 ("x"), w817, w816) -> (w811:dbl)
            n259 = Multiply(x=0.5, y=w815) -> (x*y=w814:dbl)
            n260 = control-ref of="Speed"() -> (w822:refnum<vi>)
            n261 = Select(t=w811, s=w821, f=w814) -> (s? t:f=w819:dbl)
            n262 = property class="DigNum (strict)"(reference=w822, "Value"=w819) -> ()  [unwired: 1 in, 2 out]
          }
          frame "", Default {
          }
        }
      }
      frame "ScanParameters.Send" {
        # "Be CAREFUL with NumLines which is muliplied by 2 when singleDirectionScan off"
        n263 = call "ConvertScanSizeto01.vi"("error in (no error)"=w843, "Parameters In"=w852, "Calibration"=w844) -> ("error out"=w855:errorcluster, "Parameters Out"=w854:T18)  [unwired: 4 in, 3 out]
        n264 = call "ScanparametersToFPGA.vi"("error in"=w855, "Parameters In"=w854, "FPGAIn"=w851) -> ("error out"=w857:errorcluster, "Parameters In to Send back"=w853:T18, "FPGAOut"=w850:T6)  [unwired: 4 in, 2 out]
        n265 = Unbundle By Name(w853) -> ("pointsPerLine"=w849:u32)
        n266 = call "FGVScanParameters.vi"("Enum"=Enum."Write", "error in"=w857, "Scan Parameters In"=w848) -> ("error out"=w845:errorcluster)  [unwired: 7 in, 1 out]
        n267 = Bundle By Name(cluster=w852, "pointsPerLine"=w849) -> (w846:T18)
        n268 = call "MainClusterToScanParam.vi"("error in (no error)"=w845, "Parameters Out"=w846, "Scan Parameters"=w848) -> ("error out"=w856:errorcluster)  [unwired: 8 in]
      }
      frame "ScanParameters.SendOne" {
        # "value changed 2 times"
        # "Change with an update display"
        # "Update values in the front panel if controls have a linked definition."
        n269 = Variant To Data(error in=w878, type=refnum<vi> refnum ("CtlRef"), Variant=w879) -> (data=w876:refnum<vi>, error out=w875:errorcluster)
        n270 = property class="DigNum"(reference=w876, error in=w875) -> (error out=w871:errorcluster, "Label.Text"=w874:string, "Value"=w872:variant)  [unwired: 1 out]
        n271 = Unbundle By Name(w863) -> ("Fast"=w862:dbl, "Slow"=w861:dbl)
        n272 = call "FGVScanParameters.vi"("Enum"=Enum."Read") -> ("Scan Parameters Out"=w859:T19)  [unwired: 9 in, 1 out]
        n273 = case shown="\"Time/Line\"" w874 {
          tunnel: w873 -> [w917 w935 w956 w979 w991 w1008 w1030 w1043 w1061 w1067]
          tunnel: w872 -> [w920 w937 w953 w977 w989 w1010 w1029 w1046 w1059 _]
          tunnel: [w918 w936 w954 w976 w988 w1009 w1028 w1042 w1057 w1067] -> w867
          tunnel: w871 -> [w921 w939 w957 w980 w986 w1012 _ w1044 w1060 w1066]
          tunnel: [w922 w934 w960 w967 w987 w997 w1021 w1041 w1050 w1066] -> w870
          tunnel: w862 -> [w912 _ w950 _ _ _ _ _ _ _]
          tunnel: w861 -> [_ w931 _ w973 _ _ _ _ _ _]
          tunnel: [TRUE w929 TRUE TRUE TRUE TRUE TRUE TRUE TRUE FALSE] -> w868
          tunnel: [w909 w926 w948 w970 w984 w995 w1016 w1038 w1052 w1064] -> w860
          tunnel: w859 -> [w908 w927 w947 w969 w983 w1005 w1026 w1037 w1053 w1064]
          tunnel: w880 -> [_ _ _ _ _ _ _ _ w1062 _]
          frame "Width" {
            # "Restrictions: Value of width depends on the value of offset and angle to not exceed the range"
            n274 = Unbundle By Name(w917) -> ("scanSizeSlow"=w913:dbl, "xOffset"=w900:dbl, "timePerLine"=w914:dbl)  [unwired: 1 out]
            n275 = Absolute Value(x=w900) -> (abs(x)=w899:dbl)
            n276 = Variant To Data(error in=w921, type=0.0 ("scanSizeFast"), Variant=w920) -> (data=w904:dbl, error out=w922:errorcluster)
            n277 = Add(x=w899, y=w904) -> (x+y=w907:dbl)
            n278 = In Range and Coerce(upper limit=w912, x=w907, lower limit=1e-12) -> (coerced(x)=w911:dbl)  [unwired: 1 out]
            n279 = Subtract(x=w911, y=w899) -> (x-y=w902:dbl)
            n280 = property on="Lock Scan Height" class="Bool (strict)"() -> ("Value"=w916:bool)  [unwired: 2 in, 2 out]
            n281 = Select(t=w902, s=w916, f=w913) -> (s? t:f=w910:dbl)
            n282 = Multiply(x=w902, y=2.0 ("x")) -> (x*y=w906:dbl)
            n283 = property on="Height" class="DigNum (strict)"("Value"=w910) -> ()  [unwired: 2 in, 2 out]
            n284 = property on="Width" class="DigNum (strict)"("Value"=w902) -> ()  [unwired: 2 in, 2 out]
            n285 = Divide(x=w906, y=w914) -> (x/y=w905:dbl)
            n286 = Bundle By Name(cluster=w917, "scanSizeFast"=w902, "scanSizeSlow"=w910) -> (w918:T18)
            n287 = property on="Speed" class="DigNum (strict)"("Value"=w905) -> ()  [unwired: 2 in, 2 out]
            n288 = Bundle By Name(cluster=w908, "Height"=w910, "Width"=w902) -> (w909:T19)
          }
          frame "Height" {
            # "As the height is disabled when it is locked, no need to update the width"
            n289 = property on="Y Offset" class="DigNum (strict)"() -> ("Value"=w924:dbl)  [unwired: 2 in, 2 out]
            n290 = Variant To Data(error in=w939, type=0.0 ("scanSizeFast"), Variant=w937) -> (data=w928:dbl, error out=w934:errorcluster)
            n291 = Absolute Value(x=w924) -> (abs(x)=w923:dbl)
            n292 = Add(x=w923, y=w928) -> (x+y=w932:dbl)
            n293 = In Range and Coerce(upper limit=w931, x=w932, lower limit=1e-12) -> (coerced(x)=w930:dbl)  [unwired: 1 out]
            n294 = Subtract(x=w930, y=w923) -> (x-y=w925:dbl)
            n295 = Bundle By Name(cluster=w935, "scanSizeSlow"=w925) -> (w936:T18)
            n296 = property on="Height" class="DigNum (strict)"("Value"=w925) -> ()  [unwired: 2 in, 2 out]
            n297 = Equal?(x=w925, y=w928) -> (x = y?=w929:bool)
            n298 = Bundle By Name(cluster=w927, "Height"=w925) -> (w926:T19)
          }
          frame "X Offset" {
            # "X offset case (Save Line before scan disabled to move back when enabled)"
            n299 = Variant To Data(error in=w957, type=0.0 ("scanSizeFast"), Variant=w953) -> (data=w943:dbl, error out=w958:errorcluster)
            n300 = Absolute Value(x=w943) -> (abs(x)=w946:dbl)
            n301 = property on="Width" class="DigNum (strict)"(error in=w958) -> (error out=w959:errorcluster, "Value"=w951:dbl)  [unwired: 1 in, 1 out]
            n302 = Add(x=w946, y=w951) -> (x+y=w945:dbl)
            n303 = In Range and Coerce(upper limit=w950, x=w945, lower limit=1e-12) -> (coerced(x)=w944:dbl)  [unwired: 1 out]
            n304 = Subtract(x=w944, y=w951) -> (x-y=w941:dbl)
            n305 = Sign(1:w943) -> (0:w942:dbl)
            n306 = Multiply(x=w942, y=w941) -> (x*y=w940:dbl)
            n307 = property on="X Offset" class="DigNum (strict)"(error in=w959, "Value"=w940) -> (error out=w960:errorcluster)  [unwired: 1 in, 1 out]
            n308 = Bundle By Name(cluster=w956, "xOffset"=w940) -> (w954:T18)
            n309 = Bundle By Name(cluster=w947, "X Offset"=w940) -> (w948:T19)
          }
          frame "Y Offset" {
            n310 = Variant To Data(error in=w980, type=0.0 ("scanSizeFast"), Variant=w977) -> (data=w963:dbl, error out=w968:errorcluster)
            n311 = Absolute Value(x=w963) -> (abs(x)=w966:dbl)
            n312 = property on="Height" class="DigNum (strict)"(error in=w968) -> (error out=w981:errorcluster, "Value"=w972:dbl)  [unwired: 1 in, 1 out]
            n313 = Add(x=w966, y=w972) -> (x+y=w974:dbl)
            n314 = In Range and Coerce(upper limit=w973, x=w974, lower limit=1e-12) -> (coerced(x)=w965:dbl)  [unwired: 1 out]
            n315 = Subtract(x=w965, y=w972) -> (x-y=w962:dbl)
            n316 = Sign(1:w963) -> (0:w964:dbl)
            n317 = Multiply(x=w964, y=w962) -> (x*y=w961:dbl)
            n318 = Bundle By Name(cluster=w969, "Y Offset"=w961) -> (w970:T19)
            n319 = Bundle By Name(cluster=w979, "yOffset"=w961) -> (w976:T18)
            n320 = property on="Y Offset" class="DigNum (strict)"(error in=w981, "Value"=w961) -> (error out=w967:errorcluster)  [unwired: 1 in, 1 out]
          }
          frame "Angle" {
            n321 = Variant To Data(error in=w986, type=0.0 ("scanSizeFast"), Variant=w989) -> (data=w982:dbl, error out=w987:errorcluster)
            n322 = Bundle By Name(cluster=w991, "rotation"=w982) -> (w988:T18)
            n323 = Bundle By Name(cluster=w983, "Angle"=w982) -> (w984:T19)
          }
          frame "Pixels" {
            n324 = Variant To Data(error in=w1012, type=u32 0 ("scanSizeFast"), Variant=w1010) -> (data=w1003:u32, error out=w996:errorcluster)
            n325 = Unbundle By Name(w1008) -> ("numLines"=w993:u16)
            n326 = property on="Lock Scan Lines" class="Bool (strict)"() -> ("Value"=w1006:bool)  [unwired: 2 in, 2 out]
            n327 = Select(t=w1003, s=w1006, f=w993) -> (s? t:f=w1004:u32)
            n328 = Bundle By Name(cluster=w1005, "Pixels/Line"=w1003, "Lines"=w1004) -> (w995:T19)
            n329 = property on="Lines" class="DigNum (strict)"("Val(Sgnl)"=w1004) -> ()  [unwired: 2 in, 2 out]
            n330 = call "FGVScanWaveform.vi"("Enum"=Enum."Read") -> ("scanWaveFormCtl Out"=w1001:T13)  [unwired: 9 in, 1 out]
            n331 = call "FGVScanParameters.vi"("Enum"=Enum."Write", "error in"=w996, "Scan Parameters In"=w995) -> ("error out"=w992:errorcluster)  [unwired: 7 in, 1 out]
            n332 = Unbundle By Name(w1001) -> ("fastWavePts"=w1000:u16, "slowWavePts"=w999:u16)
            n333 = Bundle By Name(cluster=w1008, "pointsPerLine"=w1003, "numLines"=w1004, "fastWavePts"=w1000, "slowWavePts"=w999) -> (w1009:T18)
            n334 = call "FGVImageArray.vi"("Enum"=Enum."Init", "error in"=w992) -> ("error out"=w997:errorcluster)  [unwired: 8 in, 1 out]
          }
          frame "Lines" {
            n335 = Variant To Data(type=u16 0 ("Lines"), Variant=w1029) -> (data=w1018:u16, error out=w1017:errorcluster)  [unwired: 1 in]
            n336 = call "FGVScanWaveform.vi"("Enum"=Enum."Read") -> ("scanWaveFormCtl Out"=w1025:T13)  [unwired: 9 in, 1 out]
            n337 = Bundle By Name(cluster=w1026, "Lines"=w1018) -> (w1016:T19)
            n338 = Unbundle By Name(w1025) -> ("slowWavePts"=w1024:u16, "fastWavePts"=w1023:u16)
            n339 = call "FGVScanParameters.vi"("Enum"=Enum."Write", "error in"=w1017, "Scan Parameters In"=w1016) -> ("error out"=w1014:errorcluster)  [unwired: 7 in, 1 out]
            n340 = flat-sequence {
              tunnel: [w1031] -> w1013
              tunnel: w1014 -> [w1031]
              frame #0 {
              }
            }
            n341 = Bundle By Name(cluster=w1030, "numLines"=w1018, "slowWavePts"=w1024, "fastWavePts"=w1023) -> (w1028:T18)
            n342 = call "FGVImageArray.vi"("Enum"=Enum."Init", "error in"=w1013) -> ("error out"=w1021:errorcluster)  [unwired: 8 in, 1 out]
          }
          frame "Time/Line" {
            # "Scan Speed Calculation"
            n343 = Variant To Data(error in=w1044, type=0.0 ("timePerLine"), Variant=w1046) -> (data=w1035:dbl, error out=w1041:errorcluster)
            n344 = Unbundle By Name(w1043) -> ("scanSizeFast"=w1033:dbl)
            n345 = Multiply(x=2.0, y=w1033) -> (x*y=w1032:dbl)
            n346 = Reciprocal(x=w1035) -> (1/x=w1036:dbl)
            n347 = Divide(x=w1032, y=w1035) -> (x/y=w1039:dbl)
            n348 = property on="Speed" class="DigNum (strict)"("Value"=w1039) -> ()  [unwired: 2 in, 2 out]
            n349 = property on="Scan Rate" class="DigNum (strict)"("Value"=w1036) -> ()  [unwired: 2 in, 2 out]
            n350 = Bundle By Name(cluster=w1043, "timePerLine"=w1035) -> (w1042:T18)
            n351 = Bundle By Name(cluster=w1037, "Time/Line"=w1035, "Scan Rate"=w1036) -> (w1038:T19)
          }
          frame "Scan Rate" {
            n352 = Variant To Data(error in=w1060, type=0.0 ("timePerLine"), Variant=w1059) -> (data=w1056:dbl, error out=w1063:errorcluster)
            n353 = Unbundle By Name(w1061) -> ("scanSizeFast"=w1048:dbl)
            n354 = Reciprocal(x=w1056) -> (1/x=w1051:dbl)
            n355 = Compound Arithmetic op=MULTIPLY(w1048, 2.0 ("x"), w1056) -> (w1054:dbl)
            n356 = property on="Speed" class="DigNum (strict)"("Value"=w1054) -> ()  [unwired: 2 in, 2 out]
            n357 = Bundle By Name(cluster=w1053, "Time/Line"=w1051) -> (w1052:T19)
            n358 = property on="Time/Line" class="DigNum (strict)"("Value"=w1051) -> ()  [unwired: 2 in, 2 out]
            n359 = Bundle By Name(cluster=w1061, "timePerLine"=w1051) -> (w1057:T18)
            n360 = call "Enqueue Message.vi"("error in"=w1063, "Message"="Speed.Update", "Queue"=w1062) -> ("error out"=w1050:errorcluster)  [unwired: 7 in, 1 out]
          }
          frame "", Default {
          }
        }
        n361 = case shown="True" w868 {
          tunnel: w870 -> [w882 w895]
          tunnel: [w882 w894] -> w869
          tunnel: w867 -> [w881 w892]
          tunnel: [w881 w893] -> w866
          tunnel: w863 -> [_ w891]
          tunnel: w865 -> [w883 w890]
          tunnel: [w883 w889] -> w864
          tunnel: w860 -> [_ w886]
          frame False {
          }
          frame True {
            n362 = call "ConvertScanSizeto01.vi"("error in (no error)"=w895, "Parameters In"=w892, "Calibration"=w891) -> ("Parameters Out"=w896:T18)  [unwired: 4 in, 4 out]
            n363 = call "FGVScanParameters.vi"("Enum"=Enum."Write", "Scan Parameters In"=w886) -> ()  [unwired: 8 in, 2 out]
            n364 = call "ScanparametersToFPGA.vi"("Parameters In"=w896, "FPGAIn"=w890) -> ("error out"=w888:errorcluster, "Parameters In to Send back"=w898:T18, "FPGAOut"=w889:T6, "timePerLineNew"=w885:dbl)  [unwired: 5 in, 1 out]
            n365 = Unbundle By Name(w898) -> ("pointsPerLine"=w897:u32)
            n366 = Bundle By Name(cluster=w892, "pointsPerLine"=w897) -> (w893:T18)
            n367 = Reciprocal(x=w885) -> (1/x=w884:dbl)
            n368 = property on="Scan Rate" class="DigNum (strict)"("Value"=w884) -> ()  [unwired: 2 in, 2 out]
            n369 = call "MainClusterToScanParam.vi"("error in (no error)"=w888, "Parameters Out"=w893) -> ("error out"=w894:errorcluster)  [unwired: 9 in]
          }
        }
      }
      frame "ScanParameters.WritetoFPGA" {
        n370 = Variant To Data(error in=w1078, type=T11 {"Sensitivity"={"Sens X"=0.0, "Sens Y"=0.0, "Sens Z"=0.0}, "Range"={"Range X"=0.0, "Range Y"=0.0, "Range Z"=0.0}, "HV gain"={"HV gain X"=0.0, "HV gain Y"=0.0, "HV gain Z"=0.0}} ("element"), Variant=w1077) -> (data=w1075:T11, error out=w1092:errorcluster)
        n371 = call "FGVScanParameters.vi"("Enum"=Enum."Write", "error in"=w1092, "Scan Parameters In"=w1080) -> ("error out"=w1093:errorcluster, "Scan Parameters Out"=w1079:T19)  [unwired: 7 in]
        n372 = Unbundle By Name(w1075) -> ("Range.Range X"=w1085:dbl, "Range.Range Y"=w1084:dbl, "Range.Range Z"=w1083:dbl)
        n373 = Bundle By Name(cluster=cluster{"Slow":dbl, "Fast":dbl, "Z":dbl} {"Slow"=0.00015, "Fast"=0.00015, "Z"=0.00015} ("Calibration"), "Slow"=w1085, "Fast"=w1084, "Z"=w1083) -> (w1074:cluster{"Slow":dbl, "Fast":dbl, "Z":dbl})
        n374 = call "ConvertScanSizeto01.vi"("error in (no error)"=w1093, "Parameters In"=w1086, "Calibration"=w1074) -> ("Parameters Out"=w1090:T18)  [unwired: 4 in, 4 out]
        n375 = call "ScanparametersToFPGA.vi"("Parameters In"=w1090, "FPGAIn"=w1087) -> ("error out"=w1094:errorcluster, "Parameters In to Send back"=w1088:T18, "FPGAOut"=w1082:T6)  [unwired: 5 in, 2 out]
        n376 = Unbundle By Name(w1088) -> ("pointsPerLine"=w1089:u32)
        n377 = Bundle By Name(cluster=w1086, "pointsPerLine"=w1089) -> (w1071:T18)
        n378 = call "MainClusterToScanParam.vi"("error in (no error)"=w1094, "Parameters Out"=w1071, "Scan Parameters"=w1079) -> ("error out"=w1069:errorcluster)  [unwired: 8 in]
        n379 = call "FGVScanParametersWaveform.vi"("Enum"=Enum."Write", "error in"=w1069, "Parameters In"=w1071) -> ("error out"=w1068:errorcluster, "Parameters Out"=w1070:T18)  [unwired: 7 in]
      }
      frame "ScanParameters.ModifyOne" {
        n380 = Variant To Data(error in=w1108, type=refnum<vi> refnum ("CtlRef"), Variant=w1110) -> (data=w1107:refnum<vi>, error out=w1102:errorcluster)
        n381 = property class="DigNum"(reference=w1107, error in=w1102) -> (reference out=w1105:refnum<vi>, error out=w1097:errorcluster, "Label.Text"=w1104:string)
        n382 = xnode "Read/Write Control"("FPGA VI Reference In"=w1098, "error in"=w1097) -> ("error out"=w1096:errorcluster, "se.p.modes.se.p.enable"=w1095:bool)  [unwired: 1 out]
        n383 = case shown="\"Lines\", \"Pixels\"" w1104 {
          tunnel: w1114 -> [w1126 w1131]
          tunnel: [w1126 w1130] -> w1113
          tunnel: w1096 -> [w1125 w1128]
          tunnel: [w1125 w1129] -> w1101
          tunnel: w1095 -> [_ w1127]
          frame "False", Default {
          }
          frame "Lines", "Pixels" {
            n384 = case shown="True" w1127 {
              tunnel: w1131 -> [w1133 w1138]
              tunnel: [w1133 w1136] -> w1130
              tunnel: [w1132 w1135] -> w1129
              tunnel: w1128 -> [w1132 w1134]
              frame False {
              }
              frame True {
                n385 = call "Enqueue Message.vi"("error in"=w1134, "Message"="Scan.Disable", "Queue"=w1138) -> ("error out"=w1135:errorcluster, "Queue dup."=w1136:refnum<queue>)  [unwired: 7 in]
              }
            }
          }
        }
        n386 = call "Enqueue Message.vi"("error in"=w1101, "Data"=w1105, "Message"="ScanParameters.SendOne", "Queue"=w1113) -> ("error out"=w1100:errorcluster, "Queue dup."=w1103:refnum<queue>)  [unwired: 6 in]
        n387 = case shown="\"Lines\", \"Pixels\"" w1104 {
          tunnel: w1103 -> [_ w1119]
          tunnel: w1100 -> [w1115 w1118]
          tunnel: [w1115 w1117] -> w1099
          tunnel: w1095 -> [_ w1116]
          frame "False", Default {
          }
          frame "Lines", "Pixels" {
            n388 = case shown="True" w1116 {
              tunnel: w1119 -> [_ w1124]
              tunnel: w1118 -> [w1120 w1122]
              tunnel: [w1120 w1121] -> w1117
              frame False {
              }
              frame True {
                n389 = call "Enqueue Message.vi"("error in"=w1122, "Message"="Scan.Enable", "Queue"=w1124) -> ("error out"=w1121:errorcluster)  [unwired: 7 in, 1 out]
              }
            }
          }
        }
      }
      frame "Speed.Update" {
        # "For the resonance compensation"
        n390 = Obtain Queue(name (unnamed)="ScanWaveforms", element data type=T12 {"Message"="", "Données de message"=variant} ("Cluster Message"), error in (no error)=w1148) -> (queue out=w1143:refnum<queue>, error out=w1142:errorcluster)  [unwired: 2 in, 1 out]
        n391 = Enqueue Element(queue=w1143, element=T12 {"Message"="Speed.Update", "Données de message"=variant} ("Cluster Message"), error in (no error)=w1142) -> (error out=w1139:errorcluster)  [unwired: 1 in, 2 out]
      }
      frame "Monitor.ScanParameters" {
        n392 = Obtain Queue(name (unnamed)="Monitor", element data type=T12 {"Message"="", "Données de message"=variant} ("Cluster Message"), error in (no error)=w1157) -> (queue out=w1158:refnum<queue>, error out=w1151:errorcluster)  [unwired: 2 in, 1 out]
        n393 = Enqueue Element(queue=w1158, element=T12 {"Message"="Parameter.Change", "Données de message"=variant} ("Cluster Message"), error in (no error)=w1151) -> (error out=w1149:errorcluster)  [unwired: 1 in, 2 out]
      }
      frame "------- Scan Waveforms -------" {
      }
      frame "ScanWaveform.Initialize" {
        # "GENERATES THE WAVEFORM and write it in the FGV"
        # "Init the waveform just once\nand save the init waveform in the cluster WaveformInit"
        n394 = Unbundle By Name(w1163) -> ("fastWavePts"=w1176:u16, "fastWaveType"=w1178:T8, "fastRoundPts"=w1179:u16, "slowWavePts"=w1175:u16, "slowWaveType"=w1177:T8, "slowRoundPts"=w1180:u16, "singleDirectionScan"=w1181:bool)
        n395 = flat-sequence {
          tunnel: w1176 -> [w1210]
          tunnel: w1178 -> [w1209]
          tunnel: w1179 -> [w1208]
          tunnel: [w1206] -> w1199
          tunnel: w1175 -> [w1206]
          tunnel: w1177 -> [w1205]
          tunnel: [w1205] -> w1198
          tunnel: [w1204] -> w1197
          tunnel: w1180 -> [w1204]
          tunnel: w1181 -> [w1203]
          tunnel: [w1203] -> w1196
          tunnel: [w1202] -> w1195
          tunnel: [w1201] -> w1173
          tunnel: w1199 -> [w1218]
          tunnel: w1198 -> [w1217]
          tunnel: w1197 -> [w1216]
          tunnel: w1196 -> [w1215]
          tunnel: w1195 -> [w1214]
          tunnel: [w1214] -> w1194
          tunnel: [w1213] -> w1193
          tunnel: w1173 -> [w1212]
          tunnel: [w1212] -> w1165
          frame #0 {
            n396 = call "scanWaveGen_deBullshitFP.vi"("overScanBlanking"=TRUE, "singleDirScan"=FALSE, "numRoundingPts"=w1208, "scanWaveForm"=w1209, "numPts"=w1210) -> ("blankingParams"=w1201:T23, "outWave"=w1202:dbl[])  [unwired: 5 in]
          }
          frame #1 {
            n397 = call "scanWaveGen_deBullshitFP.vi"("overScanBlanking"=TRUE, "singleDirScan"=w1215, "numRoundingPts"=w1216, "scanWaveForm"=w1217, "numPts"=w1218) -> ("outWave"=w1213:dbl[])  [unwired: 5 in, 1 out]
          }
        }
        n398 = Bundle By Name(cluster=T13 {"slowWavePts"=1024, "fastWavePts"=1024, "slowWaveType"=enum."Triangle", "fastWaveType"=enum."Rounded", "slowRoundPts"=8, "fastRoundPts"=32, "singleDirectionScan"=TRUE} ("scanWaveFormCtl In"), "slowWavePts"=w1175, "fastWavePts"=w1176, "slowWaveType"=w1177, "fastWaveType"=w1178, "slowRoundPts"=w1180, "fastRoundPts"=w1179, "singleDirectionScan"=w1181) -> (w1182:T13)
        n399 = call "FGVScanWaveform.vi"("Enum"=Enum."Write", "scanWaveFormCtl In"=w1182) -> ()  [unwired: 8 in, 2 out]
        n400 = call "FGVWaveformShape.vi"("Enum"=Enum."Init", "error in"=w1192, "Waveform Shape Slow In"=w1193, "Waveform Shape Fast In"=w1194) -> ("error out"=w1188:errorcluster, "WaveformInit"=w1187:T24, "Framing up? (down: f) out"=w1171:bool)  [unwired: 3 in, 2 out]
        n401 = Unbundle(w1187) -> ("Waveform Shape Fast In"=w1186:dbl[], "Waveform Shape Slow In"=w1185:dbl[])
        n402 = call "FGVWaveformShape.vi"("Framing up? (down: f) In"=w1171, "Enum"=Enum."Write", "error in"=w1188, "Waveform Shape Slow In"=w1185, "Waveform Shape Fast In"=w1186) -> ("error out"=w1167:errorcluster)  [unwired: 2 in, 4 out]
        n403 = xnode "Read/Write Control"("FPGA VI Reference In"=w1170, "error in"=w1167) -> ("FPGA VI Reference Out"=w1169:T6, "error out"=w1166:errorcluster, "se.p.clocks"=w1168:T25)
        n404 = Bundle By Name(cluster=w1168, "se.p.fastBlanking"=w1165) -> (w1164:T25)
        n405 = xnode "Read/Write Control"("FPGA VI Reference In"=w1169, "error in"=w1166, "se.p.clocks"=w1164) -> ("FPGA VI Reference Out"=w1191:T6, "error out"=w1184:errorcluster)
      }
      frame "ScanWaveform.Send" {
        # "Write point by point the X (fast) and Y (slow) waveform to the dedicated memory (FPGA)"
        # "Trying to have an execution in //"
        # "Stops the data flow towards FPGA"
        n406 = call "FGVWaveformShape.vi"("Enum"=Enum."Read", "error in"=w1238) -> ("error out"=w1242:errorcluster, "Waveform Shape Slow Out"=w1228:dbl[], "Waveform Shape Fast Out"=w1232:dbl[])  [unwired: 5 in, 2 out]
        n407 = for {
          tunnel: [w1262] -> w1234
          tunnel: [w1260] -> w1233
          tunnel: w1232 -> [w1259] mode=indexing
          tunnel: w1242 -> [w1258]
          tunnel: w1240 -> [w1257]
          tunnel: T14 {"write"=TRUE, "index"=0, "data"=0.0} ("slowWaveWrite") -> [w1256]
          i -> [w1264]
          n408 = To Unsigned Word Integer(number=w1264) -> (unsigned 16bit integer=w1255:u16)
          n409 = To Fixed-Point(number=w1259) -> (fixed-point=w1261:fxp<+/-,18,5>)  [unwired: 1 in]
          n410 = Bundle By Name(cluster=w1256, "data"=w1261, "index"=w1255) -> (w1263:T14)
          n411 = xnode "Read/Write Control"("FPGA VI Reference In"=w1257, "error in"=w1258, "se.m.fastAxis"=w1263) -> ("FPGA VI Reference Out"=w1262:T6, "error out"=w1260:errorcluster)
        }
        n412 = for {
          tunnel: [w1252] -> w1230
          tunnel: [w1250] -> w1229
          tunnel: w1242 -> [w1249]
          tunnel: w1240 -> [w1248]
          tunnel: w1228 -> [w1247] mode=indexing
          tunnel: T14 {"write"=TRUE, "index"=0, "data"=0.0} ("slowWaveWrite") -> [w1246]
          i -> [w1254]
          n413 = To Fixed-Point(number=w1247) -> (fixed-point=w1251:fxp<+/-,18,5>)  [unwired: 1 in]
          n414 = To Unsigned Word Integer(number=w1254) -> (unsigned 16bit integer=w1245:u16)
          n415 = Bundle By Name(cluster=w1246, "data"=w1251, "index"=w1245) -> (w1253:T14)
          n416 = xnode "Read/Write Control"("FPGA VI Reference In"=w1248, "error in"=w1249, "se.m.slowAxis"=w1253) -> ("FPGA VI Reference Out"=w1252:T6, "error out"=w1250:errorcluster)
        }
        n417 = xnode "Read/Write Control"("FPGA VI Reference In"=w1230, "error in"=w1229, "se.m.slowAxis"=T14 {"write"=FALSE, "index"=0, "data"=0.0} ("fastWaveWrite")) -> ("FPGA VI Reference Out"=w1239:T6, "error out"=w1243:errorcluster)
        n418 = xnode "Read/Write Control"("FPGA VI Reference In"=w1234, "error in"=w1233, "se.m.fastAxis"=T14 {"write"=FALSE, "index"=0, "data"=0.0} ("fastWaveWrite")) -> ("error out"=w1225:errorcluster)  [unwired: 1 out]
        n419 = Merge Errors(w1225, w1243) -> (w1244:errorcluster)
        n420 = Obtain Queue(name (unnamed)="ScanWaveforms", element data type=T12 {"Message"="", "Données de message"=variant} ("Cluster Message"), error in (no error)=w1244) -> (queue out=w1220:refnum<queue>, error out=w1222:errorcluster)  [unwired: 2 in, 1 out]
        n421 = call "Enqueue Message.vi"("error in"=w1222, "Message"="Refresh.Graph", "Queue"=w1220) -> ("error out"=w1221:errorcluster)  [unwired: 7 in, 1 out]
      }
      frame "XWaveform.Send" {
        n422 = call "FGVWaveformShape.vi"("Enum"=Enum."Read", "error in"=w1272) -> ("error out"=w1277:errorcluster, "Waveform Shape Fast Out"=w1273:dbl[])  [unwired: 5 in, 3 out]
        n423 = for {
          tunnel: [w1284] -> w1275
          tunnel: [w1282] -> w1274
          tunnel: w1273 -> [w1281] mode=indexing
          tunnel: w1277 -> [w1280]
          tunnel: w1269 -> [w1279]
          tunnel: T14 {"write"=TRUE, "index"=0, "data"=0.0} ("slowWaveWrite") -> [w1278]
          i -> [w1286]
          n424 = To Fixed-Point(number=w1281) -> (fixed-point=w1283:fxp<+/-,18,5>)  [unwired: 1 in]
          n425 = Bundle By Name(cluster=w1278, "data"=w1283, "index"=w1286) -> (w1285:T14)
          n426 = xnode "Read/Write Control"("FPGA VI Reference In"=w1279, "error in"=w1280, "se.m.fastAxis"=w1285) -> ("FPGA VI Reference Out"=w1284:T6, "error out"=w1282:errorcluster)
        }
        n427 = xnode "Read/Write Control"("FPGA VI Reference In"=w1275, "error in"=w1274, "se.m.fastAxis"=T14 {"write"=FALSE, "index"=0, "data"=0.0} ("fastWaveWrite")) -> ("FPGA VI Reference Out"=w1268:T6, "error out"=w1271:errorcluster)
      }
      frame "YWaveform.Send" {
        n428 = call "FGVWaveformShape.vi"("Enum"=Enum."Read", "error in"=w1292) -> ("error out"=w1291:errorcluster, "Waveform Shape Slow Out"=w1290:dbl[])  [unwired: 5 in, 3 out]
        n429 = for {
          tunnel: [w1306] -> w1298
          tunnel: [w1304] -> w1297
          tunnel: w1291 -> [w1303]
          tunnel: w1294 -> [w1302]
          tunnel: w1290 -> [w1301] mode=indexing
          tunnel: T14 {"write"=TRUE, "index"=0, "data"=0.0} ("slowWaveWrite") -> [w1300]
          i -> [w1308]
          n430 = To Fixed-Point(number=w1301) -> (fixed-point=w1305:fxp<+/-,18,5>)  [unwired: 1 in]
          n431 = Bundle By Name(cluster=w1300, "data"=w1305, "index"=w1308) -> (w1307:T14)
          n432 = xnode "Read/Write Control"("FPGA VI Reference In"=w1302, "error in"=w1303, "se.m.slowAxis"=w1307) -> ("FPGA VI Reference Out"=w1306:T6, "error out"=w1304:errorcluster)
        }
        n433 = xnode "Read/Write Control"("FPGA VI Reference In"=w1298, "error in"=w1297, "se.m.slowAxis"=T14 {"write"=FALSE, "index"=0, "data"=0.0} ("fastWaveWrite")) -> ("FPGA VI Reference Out"=w1295:T6, "error out"=w1296:errorcluster)
      }
      frame "ScanWaveforms.Update" {
        n434 = call "FGVScanWaveform.vi"("Enum"=Enum."Read", "error in"=w1323) -> ("error out"=w1311:errorcluster, "scanWaveFormCtl Out"=w1321:T13)  [unwired: 8 in]
        n435 = Unbundle By Name(w1321) -> ("slowWavePts"=w1319:u16, "fastWavePts"=w1318:u16, "slowWaveType"=w1317:T8, "fastWaveType"=w1316:T8, "slowRoundPts"=w1315:u16, "fastRoundPts"=w1314:u16)
        n436 = call "FGVScanParametersWaveform.vi"("Enum"=Enum."Read") -> ("Parameters Out"=w1320:T18)  [unwired: 9 in, 1 out]
        n437 = Bundle By Name(cluster=w1320, "slowWavePts"=w1319, "fastWavePts"=w1318, "slowWaveType"=w1317, "fastWaveType"=w1316, "slowRoundPts"=w1315, "fastRoundPts"=w1314) -> (w1313:T18)
        n438 = call "Enqueue Message.vi"("error in"=w1311, "Message"="ScanParameters.Send", "Queue"=w1312) -> ("error out"=w1309:errorcluster)  [unwired: 7 in, 1 out]
      }
      frame "--------- Scan Actions ---------" {
      }
      frame "Continuous" {
        # "Idea\nframe up/frame down already true\n- if continuous is true, single scan direction\n- if continuous is switched to false, not single scan direction"
        n439 = Variant To Data(error in=w1338, type=TRUE, Variant=w1336) -> (data=w1334:bool, error out=w1337:errorcluster)
        n440 = Not(x=w1334) -> (.not. x?=w1332:bool)
        n441 = call "Enqueue Message.vi"("error in"=w1337, "Data"=w1332, "Message"="ScanDirection.Change", "Queue"=w1342) -> ("error out"=w1341:errorcluster)  [unwired: 6 in, 1 out]
      }
      frame "Scan.Enable" {
        w1359 = TRUE ("scanEnabled")
        n442 = property on="Continuous" class="Bool (strict)"() -> ("Value"=w1348:bool)  [unwired: 2 in, 2 out]
        n443 = Not(x=w1348) -> (.not. x?=w1349:bool)
        n444 = xnode "Read/Write Control"("FPGA VI Reference In"=w1361, "error in"=w1360) -> ("FPGA VI Reference Out"=w1355:T6, "error out"=w1356:errorcluster, "se.p.modes"=w1354:T22)
        n445 = Bundle By Name(cluster=w1354, "se.mot.p.start"=TRUE ("scanEnabled"), "se.p.singleDirection"=w1349) -> (w1352:T22)
        n446 = Bundle By Name(cluster=w1362, "scanEnable"=w1359) -> (w1344:T18)
        n447 = Bundle By Name(cluster=w1352, "se.p.enable"=w1359) -> (w1353:T22)
        n448 = xnode "Read/Write Control"("FPGA VI Reference In"=w1355, "error in"=w1356, "se.p.modes"=w1352) -> ("FPGA VI Reference Out"=w1351:T6, "error out"=w1350:errorcluster)
        n449 = flat-sequence {
          tunnel: w1351 -> [w1366]
          tunnel: [w1366] -> w1364
          tunnel: [w1365] -> w1363
          tunnel: w1350 -> [w1365]
          frame #0 {
            n450 = Wait (ms)(milliseconds to wait=u32 100) -> ()  [unwired: 1 out]
          }
        }
        n451 = xnode "Read/Write Control"("FPGA VI Reference In"=w1364, "error in"=w1363, "se.p.modes"=w1353) -> ("FPGA VI Reference Out"=w1347:T6, "error out"=w1346:errorcluster)
        n452 = call "FGVScanParametersWaveform.vi"("Enum"=Enum."Write", "Parameters In"=w1344) -> ("Parameters Out"=w1343:T18)  [unwired: 8 in, 1 out]
      }
      frame "Scan.Pause" {
        n453 = property on="Pause" class="Bool (strict)"(error in=w1373) -> (error out=w1372:errorcluster, "Value"=w1371:bool)  [unwired: 1 in, 1 out]
        n454 = xnode "Read/Write Control"("FPGA VI Reference In"=w1375, "error in"=w1372) -> ("FPGA VI Reference Out"=w1379:T6, "error out"=w1378:errorcluster, "se.p.modes"=w1377:T22)
        n455 = Bundle By Name(cluster=w1377, "se.p.haltScan"=w1371) -> (w1376:T22)
        n456 = xnode "Read/Write Control"("FPGA VI Reference In"=w1379, "error in"=w1378, "se.p.modes"=w1376) -> ("FPGA VI Reference Out"=w1374:T6, "error out"=w1369:errorcluster)
      }
      frame "Scan.Disable" {
        w1385 = FALSE ("scanEnabled")
        n457 = xnode "Read/Write Control"("FPGA VI Reference In"=w1388, "error in"=w1393) -> ("FPGA VI Reference Out"=w1389:T6, "error out"=w1391:errorcluster, "se.p.modes"=w1390:T22)
        n458 = Bundle By Name(cluster=w1392, "scanEnable"=w1385) -> (w1381:T18)
        n459 = Bundle By Name(cluster=w1390, "se.p.enable"=w1385) -> (w1384:T22)
        n460 = xnode "Read/Write Control"("FPGA VI Reference In"=w1389, "error in"=w1391, "se.p.modes"=w1384) -> ("FPGA VI Reference Out"=w1383:T6, "error out"=w1387:errorcluster)
        n461 = call "FGVScanParametersWaveform.vi"("Enum"=Enum."Write", "Parameters In"=w1381) -> ("Parameters Out"=w1380:T18)  [unwired: 8 in, 1 out]
      }
      frame "From TOther VIs" {
      }
      frame "Monitor.ZoomOffset" {
        n462 = Variant To Data(error in=w1405, type=cluster{"ControlName":string, "Value":dbl} {"ControlName"="", "Value"=0.0} ("Data"), Variant=w1404) -> (data=w1400:cluster{"ControlName":string, "Value":dbl}, error out=w1403:errorcluster)
        n463 = Unbundle By Name(w1400) -> ("ControlName"=w1399:string, "Value"=w1398:dbl)
        n464 = case shown="\"Width\", Default" w1399 {
          tunnel: w1403 -> [w1411 w1414 w1417 w1420]
          tunnel: [w1410 w1413 w1416 w1419] -> w1402
          tunnel: w1398 -> [w1409 w1412 w1415 w1418]
          frame "Width", Default {
            n465 = property on="Width" class="DigNum (strict)"(error in=w1411, "Val(Sgnl)"=w1409) -> (error out=w1410:errorcluster)  [unwired: 1 in, 1 out]
          }
          frame "X Offset" {
            n466 = property on="X Offset" class="DigNum (strict)"(error in=w1414, "Val(Sgnl)"=w1412) -> (error out=w1413:errorcluster)  [unwired: 1 in, 1 out]
          }
          frame "Y Offset" {
            n467 = property on="Y Offset" class="DigNum (strict)"(error in=w1417, "Val(Sgnl)"=w1415) -> (error out=w1416:errorcluster)  [unwired: 1 in, 1 out]
          }
          frame "Height" {
            n468 = property on="Height" class="DigNum (strict)"(error in=w1420, "Val(Sgnl)"=w1418) -> (error out=w1419:errorcluster)  [unwired: 1 in, 1 out]
          }
        }
      }
      frame Default {
        w1423 = "The message \"%s\" received in the gestion loop is not valid" ("Texte de message d'erreur inconnu")
        n469 = Format Into String(format string=w1423, w1429) -> (resulting string=w1426:string)  [unwired: 2 in, 1 out]
        n470 = One Button Dialog(message=w1423, button name ("OK")="ok") -> ()  [unwired: 1 out]
        n471 = call <vilib>:"Error Cluster From Error Code.vi"("error message (\"\")"=w1426, "error code (0)"=1 ("code d'erreur (0)")) -> ("error out"=w1427:errorcluster)  [unwired: 7 in]
      }
    }
    n472 = case shown="No Error" w147 {
      selector: w147 -> [w159 w161]
      tunnel: [w159 w161] -> w146
      tunnel: [" finished" " error"] -> w145
      frame No Error {
      }
      frame Error {
      }
    }
    n473 = Concatenate Strings(w148, w145) -> (w149:string)
    n474 = local write "String"(w149) -> ()
    n475 = call "FGVScanParametersWaveform.vi"("Enum"=Enum."Write", "Parameters In"=w142) -> ()  [unwired: 8 in, 2 out]
  }
  n476 = while {
    tunnel: w15 -> [w1437]
    tunnel: [w1433] -> w14
    tunnel: w11 -> [w1432]
    tunnel: [w1431] -> w10
    stop <- w1435 stop-if-true
    # "Events loop"
    n477 = event shown="[1] \"Scan Parameters.Width\", \"Scan Parameters.Height\", \"Scan Parameters.X Offset\", \"Scan Parameters.Y Offset\", \"Scan Parameters.Angle\", \"Scan Parameters.Pixels\", \"Scan Parameters.Lines\", \"Scan Parameters.Time/Line\", \"Scan Parameters.Scan Rate\": Value Change" {
      selector: w1432 -> [_ _ _ _ _ _ _ _ _ _ _ _ _ _]
      dyn-events: [_ _ _ _ _ _ _ _ _ _ _ _ _ _] -> w1431
      timeout: 50 -> [_ _ _ _ _ _ _ _ _ _ _ _ _ _]
      tunnel: [_ _ _ _ _ _ _ _ _ _ _ w1530 _ _] -> w1436
      tunnel: w1437 -> [w1447 w1453 w1459 w1472 w1492 w1498 w1504 w1508 w1512 w1517 w1524 w1531 w1537 w1540]
      tunnel: [_ w1451 w1458 w1470 _ w1493 w1502 w1506 w1509 w1518 w1521 w1526 w1532 w1541] -> w1433
      tunnel: [w1447 w1450 w1456 w1471 w1491 w1495 w1503 w1507 w1512 w1516 w1522 w1527 w1536 w1539] -> w1434
      event Timeout {
        n478 = event-data() -> ()  [unwired: 1 in, 3 out]
      }
      event "Scan Parameters.Width", "Scan Parameters.Height", "Scan Parameters.X Offset", "Scan Parameters.Y Offset", "Scan Parameters.Angle", "Scan Parameters.Pixels", "Scan Parameters.Lines", "Scan Parameters.Time/Line", "Scan Parameters.Scan Rate": Value Change {
        n479 = event-data() -> ("CtlRef"=w1449:refnum<vi>)  [unwired: 1 in]
        n480 = To Variant(anything=w1449) -> (Variant=w1448:variant)
        n481 = call "Enqueue Message.vi"("Data"=w1448, "Message"="ScanParameters.ModifyOne", "Queue"=w1453) -> ("error out"=w1451:errorcluster, "Queue dup."=w1450:refnum<queue>)  [unwired: 7 in]
      }
      event "Lock Scan Height", "Lock Scan Lines", "Speed": Value Change {
        n482 = event-data() -> ("CtlRef"=w1455:refnum<vi>)  [unwired: 1 in]
        n483 = To Variant(anything=w1455) -> (Variant=w1454:variant)
        n484 = call "Enqueue Message.vi"("Data"=w1454, "Message"="ScanParameters.Display", "Queue"=w1459) -> ("error out"=w1458:errorcluster, "Queue dup."=w1456:refnum<queue>)  [unwired: 7 in]
      }
      event "Actions.Frame up", "Actions.Frame down", "Actions.Flip", "Actions.Stop": Mouse Down {
        # "Frame up, Frame down, Stop, Pause"
        n485 = event-data() -> ("CtlRef"=w1469:refnum<vi>)  [unwired: 1 in]
        n486 = property class="Bool"(reference=w1469) -> (reference out=w1468:refnum<vi>, "Value"=w1465:variant, "Label.Text"=w1462:string)  [unwired: 1 in, 1 out]
        n487 = Equal?(x=w1462, y="Stop") -> (x = y?=w1466:bool)
        n488 = To Variant(anything=w1468) -> (Variant=w1460:variant)
        n489 = Variant To Data(type=TRUE, Variant=w1465) -> (data=w1463:bool)  [unwired: 1 in, 1 out]
        n490 = case shown="False" w1463 {
          tunnel: w1472 -> [w1483 w1489]
          tunnel: [w1482 w1488] -> w1471
          tunnel: [w1473 w1487] -> w1470
          tunnel: w1460 -> [w1481 w1486]
          tunnel: w1466 -> [w1480 w1484]
          tunnel: w1462 -> [w1479 _]
          tunnel: "Pause" -> [w1478 _]
          frame False {
            n491 = Equal?(x=w1478, y=w1479) -> (x = y?=w1477:bool)
            n492 = Select(t="Scan.Pause" ("Message"), s=w1477, f="") -> (s? t:f=w1474:string)
            n493 = call "Enqueue Message.vi"("Prioritary message"=w1480, "Data"=w1481, "Message"=w1474, "Queue"=w1483) -> ("error out"=w1473:errorcluster, "Queue dup."=w1482:refnum<queue>)  [unwired: 6 in]
          }
          frame True {
            n494 = call "Enqueue Message.vi"("Prioritary message"=w1484, "Data"=w1486, "Message"="ScanFrame.Change", "Queue"=w1489) -> ("error out"=w1487:errorcluster, "Queue dup."=w1488:refnum<queue>)  [unwired: 6 in]
          }
        }
      }
      event "Actions.Pause": Value Change {
        n495 = event-data() -> ()  [unwired: 1 in, 1 out]
        n496 = call "Enqueue Message.vi"("Message"="Scan.Pause", "Queue"=w1492) -> ("Queue dup."=w1491:refnum<queue>)  [unwired: 8 in, 1 out]
      }
      event "Actions.Continuous": Value Change {
        n497 = event-data() -> ("NewVal"=w1497:bool)  [unwired: 1 in]
        n498 = To Variant(anything=w1497) -> (Variant=w1494:variant)
        n499 = call "Enqueue Message.vi"("Data"=w1494, "Message"="ScanDirection.Change", "Queue"=w1498) -> ("error out"=w1493:errorcluster, "Queue dup."=w1495:refnum<queue>)  [unwired: 7 in]
      }
      event "Slow scan axis": Value Change {
        n500 = event-data() -> ("NewVal"=w1500:bool)  [unwired: 1 in]
        n501 = To Variant(anything=w1500) -> (Variant=w1499:variant)
        n502 = call "Enqueue Message.vi"("Data"=w1499, "Message"="SlowScan.Disable", "Queue"=w1504) -> ("error out"=w1502:errorcluster, "Queue dup."=w1503:refnum<queue>)  [unwired: 7 in]
      }
      event "Save now": Mouse Down {
        n503 = event-data() -> ()  [unwired: 1 in, 1 out]
        n504 = call "Enqueue Message.vi"("Message"="Picture.Save", "Queue"=w1508) -> ("error out"=w1506:errorcluster, "Queue dup."=w1507:refnum<queue>)  [unwired: 8 in]
      }
      event "Auto Save": Value Change {
        n505 = event-data() -> ("NewVal"=w1510:bool)  [unwired: 1 in]
        n506 = call "FGVEndOfScan.vi"("Enum"=Enum."Write", "autoSaveIn"=w1510) -> ("error out"=w1509:errorcluster)  [unwired: 8 in, 1 out]
      }
      event "File name": Value Change {
        n507 = event-data() -> ("NewVal"=w1515:string)  [unwired: 1 in]
        n508 = To Variant(anything=w1515) -> (Variant=w1513:variant)
        n509 = call "Enqueue Message.vi"("Data"=w1513, "Message"="Filename.Update", "Queue"=w1517) -> ("error out"=w1518:errorcluster, "Queue dup."=w1516:refnum<queue>)  [unwired: 7 in]
      }
      event "Base Folder", "Exp Folder", "expno": Value Change {
        n510 = event-data() -> ()  [unwired: 1 in, 1 out]
        n511 = local read "Exp Folder"() -> (w1519:string)
        n512 = Empty String/Path?(string/path=w1519) -> (empty?=w1520:bool)
        n513 = case shown="True" w1520 {
          frame False {
          }
          frame True {
            n514 = local write "Exp Folder"("<date>_exp<#>" ("Exp Folder")) -> ()
          }
        }
        n515 = call "Enqueue Message.vi"("Message"="Folder.Update", "Queue"=w1524) -> ("error out"=w1521:errorcluster, "Queue dup."=w1522:refnum<queue>)  [unwired: 8 in]
      }
      event Panel Close? {
        w1530 = TRUE ("Rejeter ?")
        n516 = event-data() -> ()  [unwired: 1 in, 1 out]
        n517 = call "Enqueue Message.vi"("Prioritary message"=TRUE ("Message prioritaire ? (F)"), "Message"="Close", "Queue"=w1531) -> ("error out"=w1526:errorcluster, "Queue dup."=w1527:refnum<queue>)  [unwired: 7 in]
        n518 = event-data ("Event Filter Node")("Discard?"=w1530) -> ()  [unwired: 1 in, 1 out]
      }
      event Value Change {
        n519 = event-data() -> ("CtlRef"=w1535:refnum<vi>)  [unwired: 1 in]
        n520 = To Variant(anything=w1535) -> (Variant=w1533:variant)
        n521 = call "Enqueue Message.vi"("Data"=w1533, "Message"="UserEvents.Calibration", "Queue"=w1537) -> ("error out"=w1532:errorcluster, "Queue dup."=w1536:refnum<queue>)  [unwired: 7 in]
      }
      event Value Change {
        n522 = event-data() -> ("NewVal"=w1543:T27)  [unwired: 1 in]
        n523 = To Variant(anything=w1543) -> (Variant=w1542:variant)
        n524 = call "Enqueue Message.vi"("Data"=w1542, "Message"="UserEvents.ScanWaveform", "Queue"=w1540) -> ("error out"=w1541:errorcluster, "Queue dup."=w1539:refnum<queue>)  [unwired: 7 in]
      }
    }
    n525 = case shown="Error" w1433 {
      tunnel: [w1438 TRUE ("Rejeter ?")] -> w1435
      tunnel: w1436 -> [w1438 _]
      tunnel: w1434 -> [_ w1445]
      frame No Error {
      }
      frame Error {
        n526 = call "Enqueue Message.vi"("Prioritary message"=TRUE ("Message prioritaire ? (F)"), "Message"="Scan.Disable", "Queue"=w1445) -> ("error out"=w1443:errorcluster, "Queue dup."=w1442:refnum<queue>)  [unwired: 7 in]
        n527 = call "Enqueue Message.vi"("Prioritary message"=TRUE ("Message prioritaire ? (F)"), "error in"=w1443, "Message"="Exit", "Queue"=w1442) -> ()  [unwired: 6 in, 2 out]
      }
    }
  }
  n528 = Unregister For Events(event registration refnum=w10, error in=w14) -> (error out=w9:errorcluster)
  n529 = Close Reference(reference=w8, error in (no error)=w9) -> (error out=w6:errorcluster)
  n530 = Close Reference(reference=w5, error in (no error)=w6) -> (error out=w4:errorcluster)
  n531 = Merge Errors(w4, w16) -> (w1:errorcluster)
  n532 = disable-structure shown="Disabled" {
    disable-tunnel: w13 -> [w1545 _]
    disable-tunnel: w1 -> [w1544 _]
    frame Disabled {
      n533 = xnode "Close FPGA VI Reference"("FPGA VI Reference In"=w1545, "error in"=w1544) -> ()  [unwired: 1 out]
    }
    frame Enabled {
    }
  }
  n534 = flat-sequence {
    tunnel: w1 -> [w1546]
    frame #0 {
      n535 = call "FGVImageArray.vi"("Enum"=Enum."Read", "error in"=w1546) -> ("ImageRefOut"=w1547:refnum<data-value>[][])  [unwired: 8 in, 1 out]
      n536 = for {
        tunnel: w1547 -> [w1549] mode=indexing
        n537 = for {
          tunnel: w1549 -> [w1550] mode=indexing
          n538 = Delete Data Value Reference(data value reference=w1550) -> ()  [unwired: 1 in, 2 out]
        }
      }
    }
    frame #1 {
      n539 = Request Deallocation(TRUE ("flag")) -> ()
    }
  }
